vi "CP FES Walking.vi"() -> ()   [LabVIEW 2019]
uses:
  Lee Lab/CP FES Walking 2018/Code/Working/LabVIEW/Controls/Messages/Timer Messages.ctl
  Controls/Messages/CP FES Message.ctl
  <extravilib>/ChannelInstances/Messenger-t'Timer Messages.ctl'.lvlib
  Controls/Protocol Interval.ctl
  Lee Lab/CP FES Walking 2018/Code/Working/LabVIEW/Controls/States/Timer States.ctl
  <extravilib>/ChannelInstances/Event Messenger-bool.lvlib
  Controls/States/CP FES State.ctl
  Controls/Stim Interval Mode.ctl
  <extravilib>/ChannelInstances/Event Messenger-bool/Event Data.ctl
  Controls/Timer Data for timer.ctl
  Controls/Stimulator Mode.ctl
  Controls/Type Defs/Stimulator Control.ctl
  Controls/Type Defs/Stimulator Controls.ctl
  Controls/Interval on-off indicator.ctl
  Controls/Interval Array.ctl
  Controls/Protocol Cluster.ctl
  Controls/APDM Init Cluster.ctl
  Controls/GPD Side Parameters.ctl
  Controls/Stim off-half-ful.ctl
  Controls/Type Defs/Stim Parameters.ctl
  Controls/Subject Params.ctl
  Controls/CP FES Walking Data.ctl
  Controls/Subject.ctl
  Version 2/States/Protocol Timer States.ctl
  Version 2/Data Type Defs/Stim Status.ctl
  Version 2/Data Type Defs/Pulse Mode (array).ctl
  Version 2/Data Type Defs/Stim Update Data.ctl
  Version 2/Data Type Defs/Stim Init Data.ctl
  Version 2/Data Type Defs/Stim Open Data.ctl
  Version 2/Data Type Defs/Stimulator.ctl
  Controls/GPD Parameter Names.ctl
  Controls/APDM Control.ctl
  Controls/Gyro Control.ctl
  Controls/Gyro Controls.ctl
panel:
  in  "View Edit Params":bool
  in  "Thresholding":bool
  in  "Param Ctrls":T1
  out "Iteration Time (ms)":u32
  out "New remaining session time":u32
  out "New time elapsed in current iteration 2":u32
  out "New time to next interval 2":u32
  out "Current interval index 2":u32
  out "Timer State":T2(ring)
  in  "Subject":T3 items=["", "Subject 1", "Subject 2", "Subject 3", "Subject 4", "Subject 5", "Subject 6", "Subject 7", "Subject 8", "Subject 9", "Subject 10", "Subject 11", "Subject 12", "Subject 13", "Subject 14", "Subject 15", "Subject 16", "Subject 17", "Subject 18", "Subject 19", "Subject 20", "Subject 21", "Subject 22", "Subject 23", "Subject 24", "Subject 25", "Subject 26", "Subject 27", "Subject 28", "Subject 29", "Subject 30", "Subject 31", "Subject 32", "Subject 33", "Subject 34", "Subject 35", "Subject 36", "Subject 37", "Subject 38", "Subject 39"]
  in  "Tab Control":T4(tab)
  in  "APDM Hardware":T5
  in  "Protocol":T8={"Active Interval"=[], "Protocol"=[{"Interval Type"=enum."Walk", "Duration"=20.0, " Mode"=enum."Stim", "Alt Period"=0.0}, {"Interval Type"=enum."Rest", "Duration"=20.0, " Mode"=enum."No Stim", "Alt Period"=0.0}, {"Interval Type"=enum."Walk", "Duration"=20.0, " Mode"=enum."Stim", "Alt Period"=0.0}, {"Interval Type"=enum."Rest", "Duration"=20.0, " Mode"=enum."No Stim", "Alt Period"=0.0}, {"Interval Type"=enum."Walk", "Duration"=20.0, " Mode"=enum."Stim", "Alt Period"=0.0}, {"Interval Type"=enum."Rest", "Duration"=20.0, " Mode"=enum."No Stim", "Alt Period"=0.0}, {"Interval Type"=enum."Walk", "Duration"=20.0, " Mode"=enum."Stim", "Alt Period"=0.0}, {"Interval Type"=enum."Rest", "Duration"=20.0, " Mode"=enum."No Stim", "Alt Period"=0.0}, {"Interval Type"=enum."Walk", "Duration"=20.0, " Mode"=enum."Alternating", "Alt Period"=0.0}]}
  in  "Stimulators":T13={"Cluster"={"String 5"="Side", "String"="Stimulator Name", "String 2"="OK", "String 3"="Mode", "String 4"="Timeout (ms)"}, "Left Stimulator Control"={"Side"=enum."Left", "Name"="", "Open"=FALSE, " Mode"="LIVE", "Visa Timeout"=50.0}, "Right Stimulator Control"={"Side"=enum."Right", "Name"="", "Open"=FALSE, " Mode"="LIVE", "Visa Timeout"=50.0}}
  out "GPD Parameter Names":T16=["% Cycle Delay", "Min % Cycle LR to ISw ", "Min % Cycle LR to MSw", "Min % Cycle LR to TSw", "Min % Cycle ISw to MSw", "Min % Cycle TSw to LR", "Max % Cycle TSw to LR", "LR Min Gyro Z Threshold", "LR Min Gyro Z Width", "ISw Peak Threshold", "ISw Peak Width (ms)", "TSw Valley Threshold", "TSw Valley Width (ms)", "Max Cycle Time (s)", "Mean Computation Window"]
  out "GPD Params Display":T18={"Left GPD Params"={"% Cycle Delay"=75.0, "Min % Cycle LR to ISw "=55.0, "Min % Cycle LR to MSw"=50.0, "Min % Cycle LR to TSw"=75.0, "Max % Cycle ISw to MSw"=25.0, "Min % Cycle TSw to LR"=2.5, "Max % Cycle TSw to LR"=75.0, "LR Min Gyro Z Threshold"=-0.3, "LR Min Gyro Z Width"=230.0, "ISw Peak Threshold"=0.6, "ISw Peak Width"=55.0, "TSw Valley Threshold"=-0.5, "TSw Valley Width (ms)"=55.0, "Max Cycle Time (s)"=1.3, "Mean Computation Window"=10.0, "CP subject?"=FALSE}, "Right GPD Params"={"% Cycle Delay"=75.0, "Min % Cycle LR to ISw "=55.0, "Min % Cycle LR to MSw"=50.0, "Min % Cycle LR to TSw"=75.0, "Max % Cycle ISw to MSw"=25.0, "Min % Cycle TSw to LR"=2.5, "Max % Cycle TSw to LR"=75.0, "LR Min Gyro Z Threshold"=-0.3, "LR Min Gyro Z Width"=230.0, "ISw Peak Threshold"=0.6, "ISw Peak Width"=55.0, "TSw Valley Threshold"=-0.5, "TSw Valley Width (ms)"=55.0, "Max Cycle Time (s)"=1.3, "Mean Computation Window"=10.0, "CP subject?"=FALSE}}
  out "Parameters File":string
  out "Stim Params Display":T21
  out "Parameters File":string
  in  "Local Default Parameters File":path=path "\\\\win.udel.edu\\PT/Lee Lab/CP FES Walking 2018"
  out "Timer State":T2(ring)
  out "Iteration Time (ms)":u32
  out "New remaining session time":u32
  out "New time elapsed in current iteration":u32
  out "New time to next interval":u32
  out "Current interval index":u32
  in  "Subject Parameters Folder":path=path "\\\\win.udel.edu\\PT/Lee Lab/CP FES Walking 2018/Subject Parameters"
  in  "Gyro Mode":string(combo)="REAL LIVE GYRO"
  out "Source Parameter File":path
  in  "Stop GPD":bool
  in  "Start GPD":bool
  in  "Start Timer":bool
  in  "Reset":bool
  in  "Manual Stim":bool
  in  "Pause":bool
  in  "Stop":bool
  out "Session Time":dbl[unit] caption="Session Time (s)" format="%.1f"
  out "Time to Next Interval":dbl[unit] caption="Interval Time (s)" format="%.1f"
  # "Save new parameters in new file, load latest version every time"
  # "Present list of all saved parameter files"
  # "Add bluetooth app"
  # "Do an APDM hardware check before allowing Start GPD"
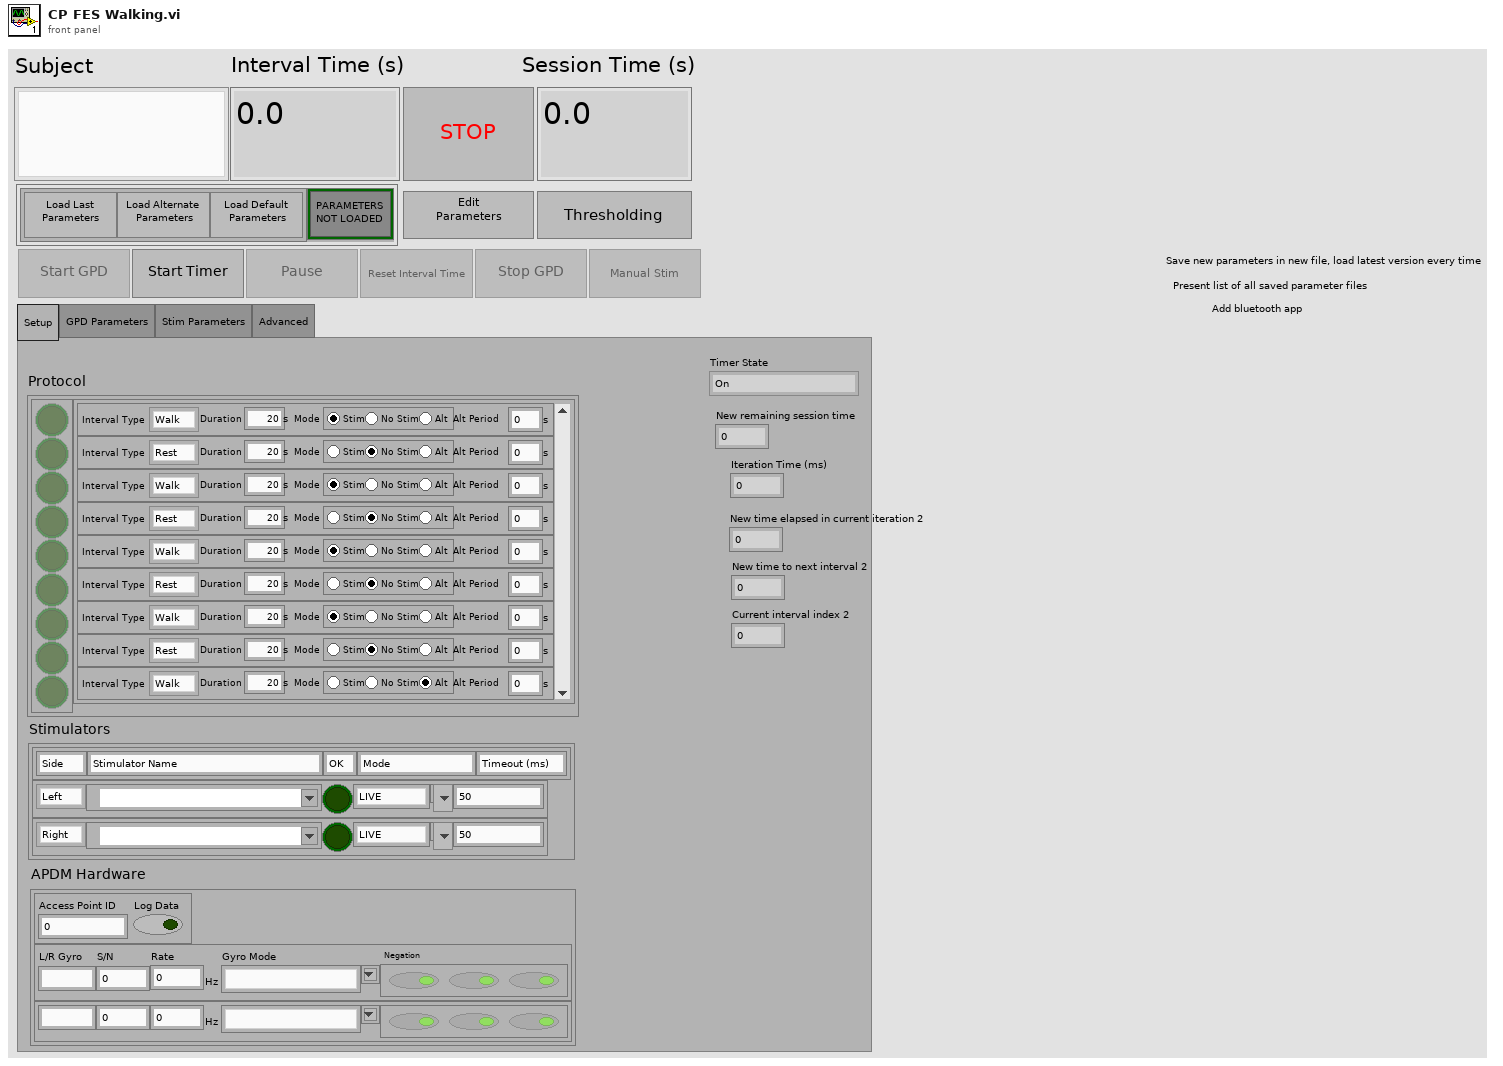
[diagram p1: front panel]
types:
  T1 = cluster{"Param Ctrls":cluster{"Load Last Parameters":bool, "Load Alternate Parameters":bool, "Load Default Parameters":bool}, "Parameters Loaded?":bool}
  T2 = enum16{"On", "Stop", "Pause", "Resume", "Idle", "Initialize"}
  T3 = typedef "Subject.ctl" = u16
  T4 = enum32{"Setup", "GPD Parameters", "Stim Parameters", "Advanced"}
  T5 = typedef "Gyro Controls.ctl" = cluster{"AP Control":T6, "Gyro Control":T7, "Gyro Control 2":T7}
  T6 = typedef "APDM Control.ctl" = cluster{"Access Point ID":u32, "Log Data":bool}
  T7 = typedef "Gyro Control.ctl" = cluster{"L/R":string, "S/N":u32, "Rate":dbl[unit], "Gyro Mode":string, " Negation":bool[]}
  T8 = typedef "Protocol Cluster.ctl" = cluster{"Active Interval":T9[], "Protocol":T10}
  T9 = typedef "Interval on-off indicator.ctl" = bool
  T10 = typedef "Interval Array.ctl" = T11[]
  T11 = typedef "Protocol Interval.ctl" = cluster{"Interval Type":enum16{"Walk", "Rest"}, "Duration":dbl[unit], " Mode":T12, "Alt Period":dbl[unit]}
  T12 = typedef "Stim Interval Mode.ctl" = enum32{"Stim", "No Stim", "Alternating"}
  T13 = typedef "Stimulator Controls.ctl" = cluster{"Cluster":cluster{"String 5":string, "String":string, "String 2":string, "String 3":string, "String 4":string}, "Left Stimulator Control":T14, "Right Stimulator Control":T14}
  T14 = typedef "Stimulator Control.ctl" = cluster{"Side":enum16{"Left", "Right"}, "Name":refnum<visa-resource-name>, "Open":bool, " Mode":T15, "Visa Timeout":dbl}
  T15 = typedef "Stimulator Mode.ctl" = string
  T16 = typedef "GPD Parameter Names.ctl" = string[]
  T17 = typedef "GPD Side Parameters.ctl" = cluster{"% Cycle Delay":dbl, "Min % Cycle LR to ISw ":dbl, "Min % Cycle LR to MSw":dbl, "Min % Cycle LR to TSw":dbl, "Max % Cycle ISw to MSw":dbl, "Min % Cycle TSw to LR":dbl, "Max % Cycle TSw to LR":dbl, "LR Min Gyro Z Threshold":dbl, "LR Min Gyro Z Width":dbl, "ISw Peak Threshold":dbl, "ISw Peak Width":dbl, "TSw Valley Threshold":dbl, "TSw Valley Width (ms)":dbl, "Max Cycle Time (s)":dbl, "Mean Computation Window":dbl, "CP subject?":bool}
  T18 = cluster{"Left GPD Params":T17, "Right GPD Params":T17}
  T19 = typedef "Stim Parameters.ctl" = cluster{"Stim Pattern Values":T20[][], "Pulse Duration":i64[], "Current":i64[]}
  T20 = typedef "Stim off-half-ful.ctl" = enum16{"Off", "Half", "Full"}
  T21 = cluster{"Left Stim Params":T19, "Right Stim Params":T19}
  T22 = typedef "Subject Params.ctl" = cluster{"Subject":T3, "Left GPD Params":T17, "Right GPD Params":T17, "Left Stim Params":T19, "Right Stim Params":T19, "Left Train length":i64[], "Right Train length":i64[]}
  T23 = typedef "APDM Init Cluster.ctl" = cluster{"Log Data":bool, "Gyro Mode":string, "Left  OPAL ID":u32, "Right OPAL ID":u32, "Access Point ID":u32}
  T24 = cluster{"Subject":u16, "Subject Parameter File":path, "Subject Parameters":T22, "Current Interval Idx":i32, "Protocol":T8, "Stimulator Controls":T13, "Stim Protocol Log File":path, "APDM Init Cluster":T23}
  T25 = cluster{"Session Over":refnum<event-registration>, "Interval Over":refnum<event-registration>}
  T26 = typedef "CP FES Message.ctl" = cluster{"State":T27, "Data":variant}
  T27 = typedef "CP FES State.ctl" = enum16{"On", "Stop", "Idle", "Initialize", "Manual", "Stim On", "Stim Off", "Start Timer", "Pause", "Resume", "Reset"}
  T28 = enum8{"Enabled", "Disabled", "Disabled and Grayed Out"}
  T29 = typedef "Timer Data for timer.ctl" = cluster{"Protocol Timer State":T30, "Remaining session time":dbl[unit], "Curent interval duration":dbl[unit], "Time of last iteration":dbl[unit], "Time elapsed in current iteration":dbl[unit], "Current interval indicator":bool[], "Current interval index":u32, "Time to next interval":dbl[unit], "Protocol":T11[]}
  T30 = typedef "Protocol Timer States.ctl" = enum16{"Initialize", "Start", "Advance", "Stop", "Pause", "Resume", "Reset"}
  T31 = typedef "Timer Messages.ctl" = cluster{"Message":T32, "Data":variant}
  T32 = typedef "Timer States.ctl" = enum16{"On", "Stop", "Pause", "Resume", "Idle", "Initialize", "Transition", "Reset", "Start"}
  T33 = typedef "Messenger-t'Timer Messages.ctl'.lvlib/))Channel.ctl" = refnum<queue>
  T34 = typedef "Event Messenger-bool.lvlib/))Channel.ctl" = refnum<queue>
  T35 = typedef "Protocol Cluster.ctl" = cluster{"Active Interval":T9[], "Protocol":T36}
  T36 = typedef "Interval Array.ctl" = T37[]
  T37 = typedef "Protocol Interval.ctl" = cluster{"Interval Type":enum16{"Walk", "Rest"}, "Duration":dbl, "Stim Mode":T12, "Alt Period":dbl}
  T38 = cluster{"Subject Parameter File":path, "Current Interval":T11, "Stim Protocol Log File":path}
  T39 = typedef "CP FES Walking Data.ctl" = cluster{"Subject":u16, "Subject Parameter File":path, "Subject Parameters":T22, "Current Interval Idx":i32, "Protocol":T8, "Stim Protocol Log File":path, "APDM Init Cluster":T23, "Stimulators":T40[]}
  T40 = typedef "Stimulator.ctl" = cluster{"Stim Open Data":T41, "Stim Init Data":T42, "Stim Update Data":T43, "Stim Status":T45}
  T41 = typedef "Stim Open Data.ctl" = cluster{"Name":refnum<visa-resource-name>, "Mode":enum16{"LIVE", "SIM"}, "Visa Timeout":u32}
  T42 = typedef "Stim Init Data.ctl" = cluster{"Frequency":dbl, "N Factor":u8, "D/T Int":dbl, "Active Channels":bool[], "LF Channels":bool[]}
  T43 = typedef "Stim Update Data.ctl" = cluster{"Pulse Mode":T44, "Current":u32[], "Pulse Dur":u32[]}
  T44 = typedef "Pulse Mode (array).ctl" = enum16{"Single", "Doublet", "Triplet"}[]
  T45 = typedef "Stim Status.ctl" = cluster{"Open":bool, "On":bool}
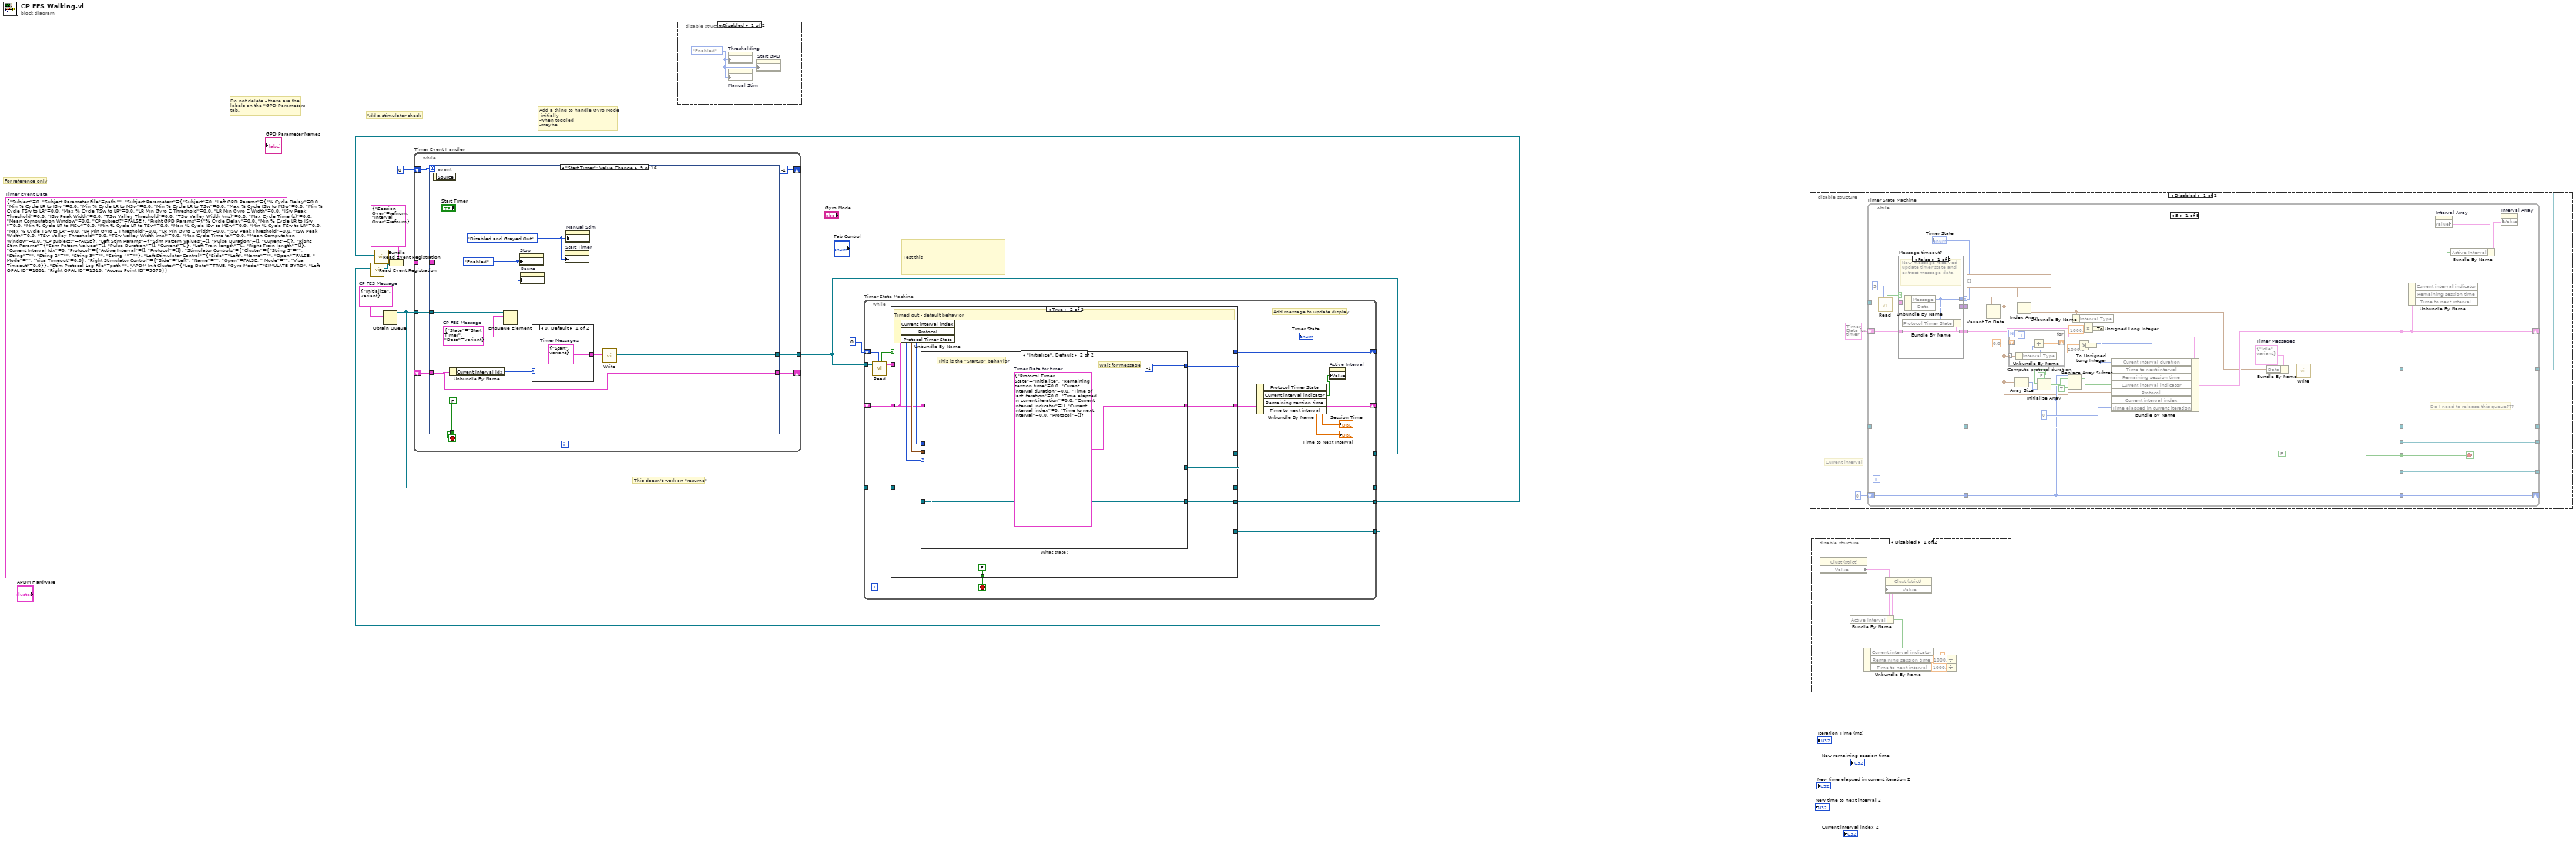
[diagram p0: block diagram]
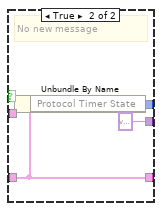
[diagram p3: hidden frame]
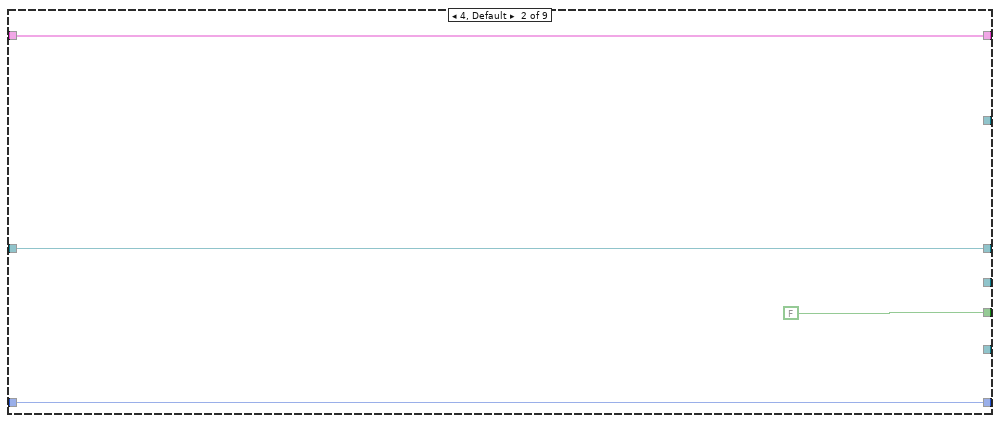
[diagram p4: hidden frame]
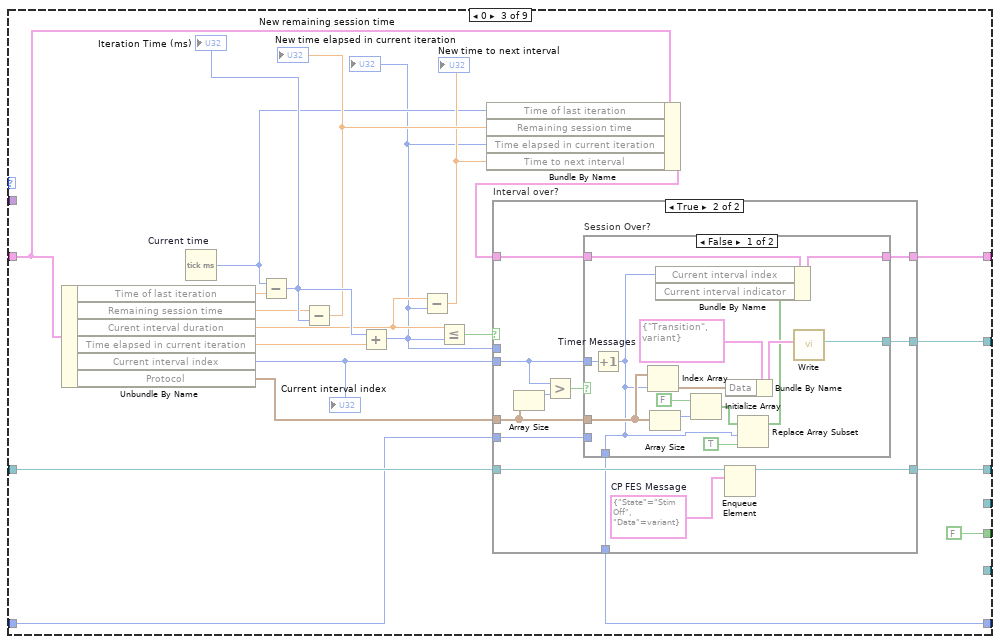
[diagram p5: hidden frame]
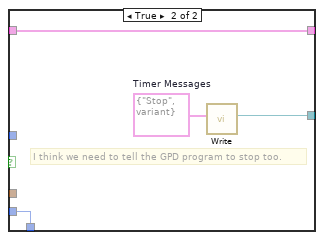
[diagram p7: hidden frame]
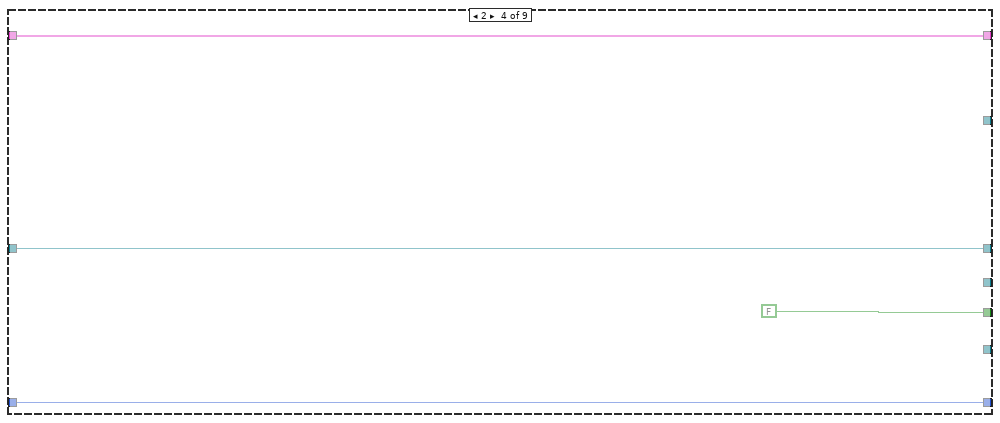
[diagram p8: hidden frame]
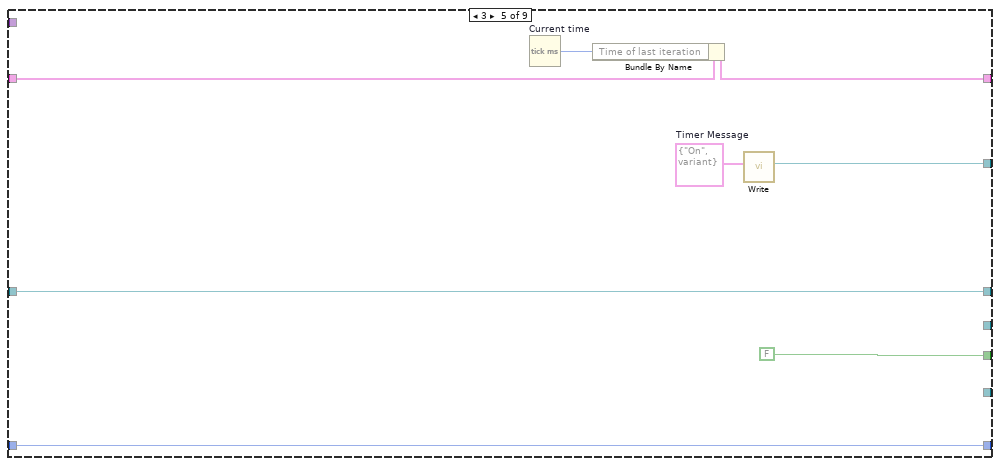
[diagram p9: hidden frame]
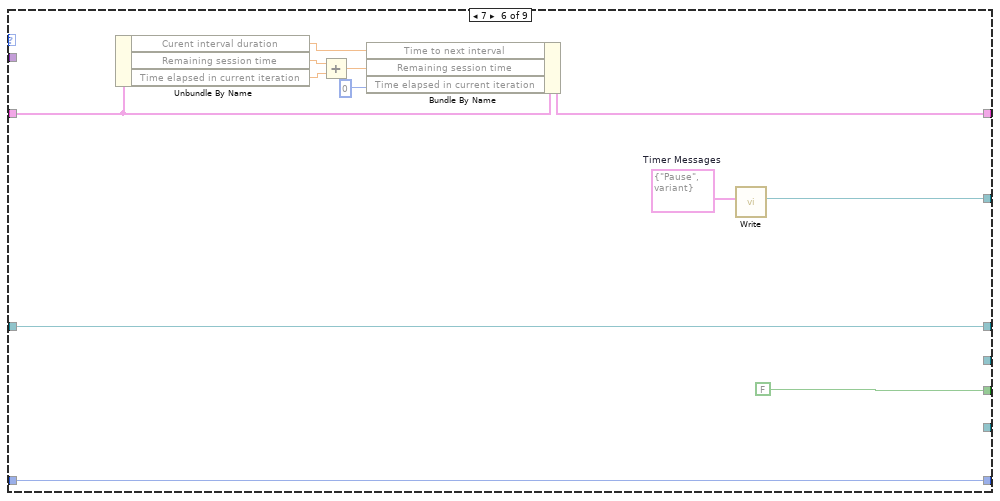
[diagram p10: hidden frame]
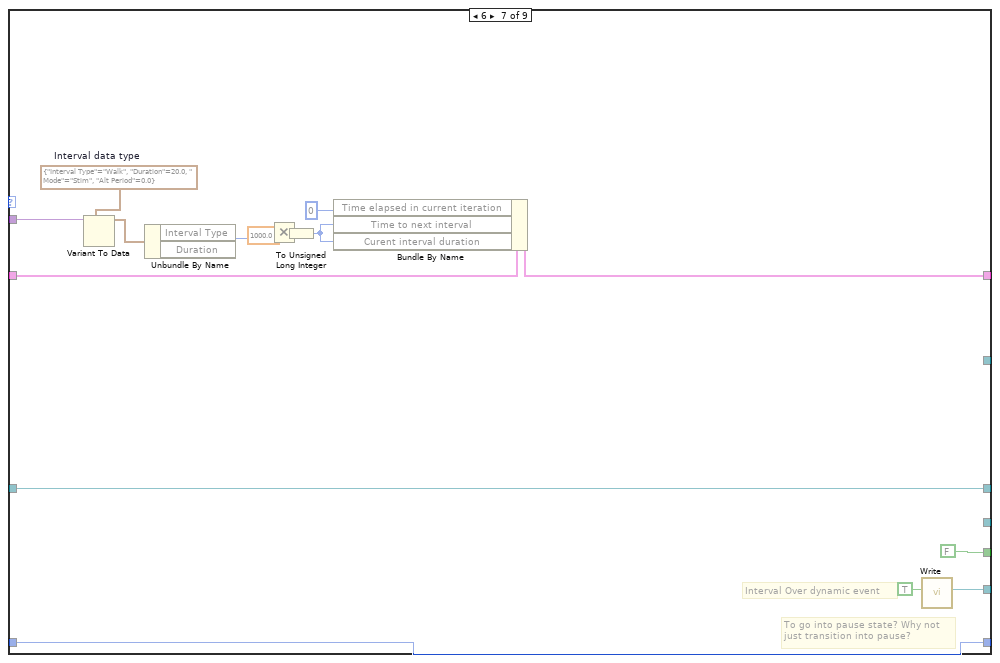
[diagram p11: hidden frame]
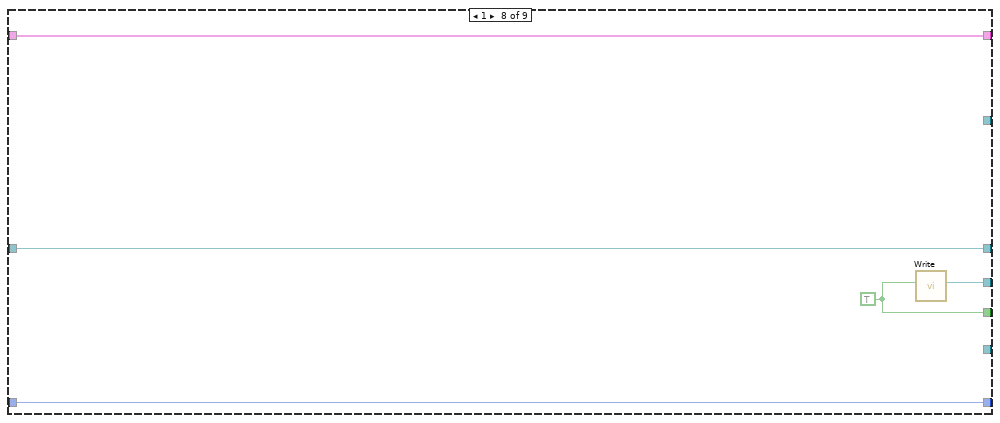
[diagram p12: hidden frame]
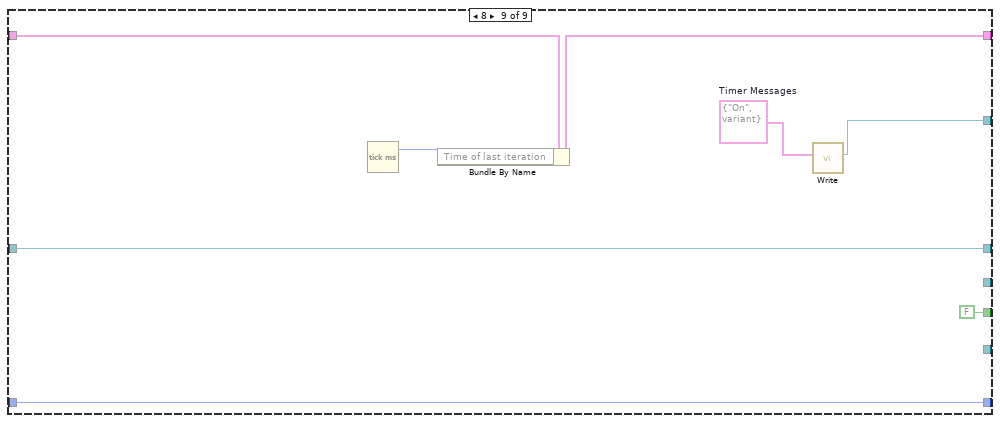
[diagram p13: hidden frame]
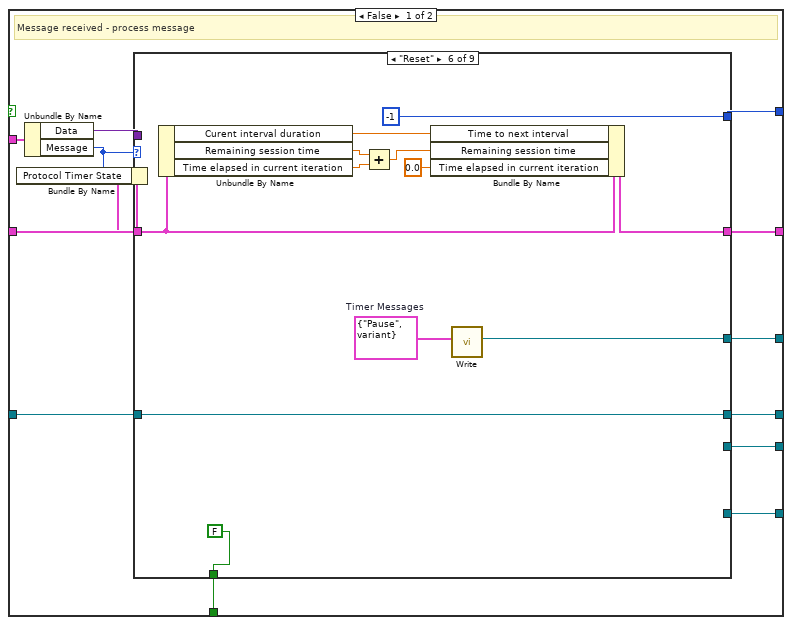
[diagram p16: hidden frame]
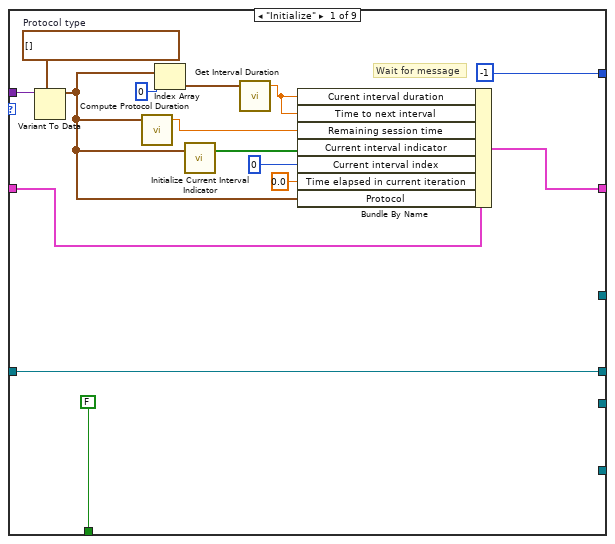
[diagram p17: hidden frame]
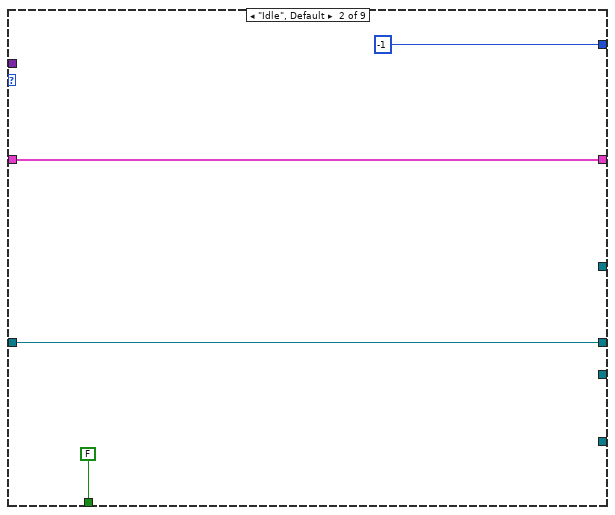
[diagram p18: hidden frame]
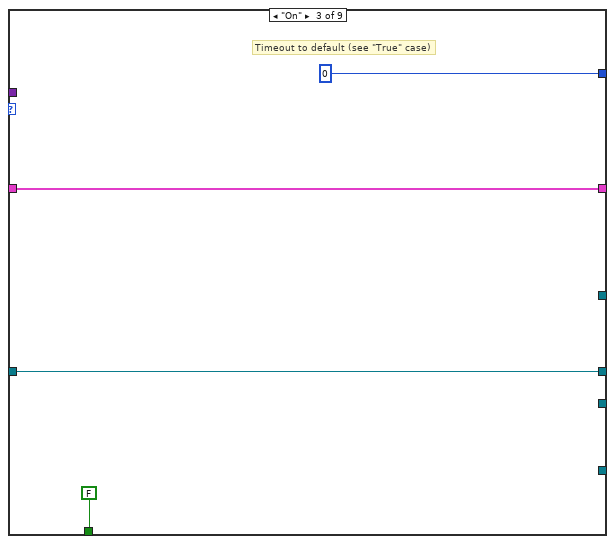
[diagram p19: hidden frame]
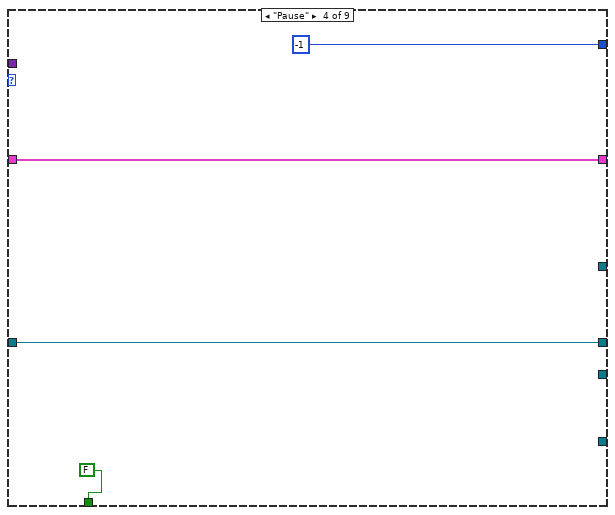
[diagram p20: hidden frame]
diagram:
  (unwired) T24 {"Subject"=0, "Subject Parameter File"=path "", "Subject Parameters"={"Subject"=0, "Left GPD Params"={"% Cycle Delay"=0.0, "Min % Cycle LR to ISw "=0.0, "Min % Cycle LR to MSw"=0.0, "Min % Cycle LR to TSw"=0.0, "Max % Cycle ISw to MSw"=0.0, "Min % Cycle TSw to LR"=0.0, "Max % Cycle TSw to LR"=0.0, "LR Min Gyro Z Threshold"=0.0, "LR Min Gyro Z Width"=0.0, "ISw Peak Threshold"=0.0, "ISw Peak Width"=0.0, "TSw Valley Threshold"=0.0, "TSw Valley Width (ms)"=0.0, "Max Cycle Time (s)"=0.0, "Mean Computation Window"=0.0, "CP subject?"=FALSE}, "Right GPD Params"={"% Cycle Delay"=0.0, "Min % Cycle LR to ISw "=0.0, "Min % Cycle LR to MSw"=0.0, "Min % Cycle LR to TSw"=0.0, "Max % Cycle ISw to MSw"=0.0, "Min % Cycle TSw to LR"=0.0, "Max % Cycle TSw to LR"=0.0, "LR Min Gyro Z Threshold"=0.0, "LR Min Gyro Z Width"=0.0, "ISw Peak Threshold"=0.0, "ISw Peak Width"=0.0, "TSw Valley Threshold"=0.0, "TSw Valley Width (ms)"=0.0, "Max Cycle Time (s)"=0.0, "Mean Computation Window"=0.0, "CP subject?"=FALSE}, "Left Stim Params"={"Stim Pattern Values"=[], "Pulse Duration"=[], "Current"=[]}, "Right Stim Params"={"Stim Pattern Values"=[], "Pulse Duration"=[], "Current"=[]}, "Left Train length"=[], "Right Train length"=[]}, "Current Interval Idx"=0, "Protocol"={"Active Interval"=[], "Protocol"=[]}, "Stimulator Controls"={"Cluster"={"String 5"="", "String"="", "String 2"="", "String 3"="", "String 4"=""}, "Left Stimulator Control"={"Side"=enum."Left", "Name"="", "Open"=FALSE, " Mode"="", "Visa Timeout"=0.0}, "Right Stimulator Control"={"Side"=enum."Left", "Name"="", "Open"=FALSE, " Mode"="", "Visa Timeout"=0.0}}, "Stim Protocol Log File"=path "", "APDM Init Cluster"={"Log Data"=TRUE, "Gyro Mode"="SIMULATE GYRO", "Left  OPAL ID"=1801, "Right OPAL ID"=1510, "Access Point ID"=9370}}  # Timer Event Data
  w11 = T26 {"State"=enum."Initialize", "Data"=variant}  # CP FES Message
  # "Do not delete - these are the\nlabels on the \"GPD Parameters\ntab."
  # "For reference only"
  # "This doesn't work on \"resume\""
  # "Test this"
  # "Add a thing to handle Gyro Mode\n-initially\n-when toggled\n-maybe"
  # "Add a stimulator check"
  n1 = Obtain Queue(element data type=w11) -> (queue out=w1:refnum<queue>)  [unwired: 4 in, 2 out]
  n2 = disable-structure shown="Disabled" {
    frame Disabled {
      w12 = T28."Enabled" ("Disabled")
      n3 = property on="Thresholding" class="Bool"("DisabledEnum"=w12) -> ()  [unwired: 2 in, 2 out]
      n4 = property on="Manual Stim" class="Bool (strict)"("DisabledEnum"=w12) -> ()  [unwired: 2 in, 2 out]
      n5 = property on="Start GPD" class="Bool"("DisabledEnum"=w12) -> ()  [unwired: 2 in, 2 out]
    }
    frame Enabled {
    }
  }
  n6 = disable-structure shown="Disabled" {
    frame Disabled {
      # "Current interval"
      n7 = while "Timer State Machine" {
        tunnel: w13 -> [w37]
        tunnel: [w32] -> w13
        shift-right: [w28] -> _
        shift-left: T29 {"Protocol Timer State"=enum."Initialize", "Remaining session time"=0.0, "Curent interval duration"=0.0, "Time of last iteration"=0.0, "Time elapsed in current iteration"=0.0, "Current interval indicator"=[], "Current interval index"=0, "Time to next interval"=0.0, "Protocol"=[]} -> [w30]
        tunnel: [w26] -> _
        tunnel: [w25] -> w15
        tunnel: [w24] -> _
        tunnel: [w23] -> _
        shift-right: [w22] -> _
        shift-left: u32 0 -> [w21]
        stop <- w34 stop-if-true
        # "Do I need to release this queue???"
        n8 = call <extravilib>:"Read.vi"("timeout in ms (-1)"=5, "channel"=w37) -> ("element"=w36:T31, "timedout?"=w31:bool)  [unwired: 6 in, 2 out]
        n9 = case "Message timeout?" shown="False" w31 {
          tunnel: w36 -> [w42 _]
          tunnel: [w40 w43] -> w35
          tunnel: [w41 variant ("Data")] -> w33
          tunnel: w30 -> [w39 w44]
          tunnel: [w38 w44] -> w29
          frame False {
            # "New message received - update timer state and extract message data"
            n10 = Unbundle By Name(w42) -> ("Message"=w40:T32, "Data"=w41:variant)
            n11 = Bundle By Name(cluster=w39, "Protocol Timer State"=w40) -> (w38:T29)
          }
          frame True {
            # "No new message"
            n12 = Unbundle By Name(w44) -> ("Protocol Timer State"=w43:T30)
          }
        }
        "Timer State" <- w35
        n13 = case shown="5" w35 {
          tunnel: [FALSE FALSE FALSE FALSE FALSE FALSE FALSE w177 FALSE] -> w34
          tunnel: w33 -> [w69 _ _ _ _ _ w172 _ _]
          tunnel: [w67 _ w100 _ w144 w156 _ _ w183] -> w32
          tunnel: w29 -> [w58 w79 w92 w137 w143 w153 w167 w178 w185]
          tunnel: [w53 w79 w88 w137 w141 w150 w166 w178 w184] -> w28
          tunnel: [_ _ _ _ _ _ _ w176 _] -> w26
          tunnel: w25 -> [w50 w78 w86 w136 w140 w149 w160 w175 w181]
          tunnel: [w50 w78 w83 w136 w140 w149 w160 w175 w181] -> w24
          tunnel: [_ _ _ _ _ _ w161 _ _] -> w23
          tunnel: [w48 w77 w82 w135 w139 w148 w159 w174 w180] -> w22
          tunnel: w21 -> [w48 w77 w81 w135 w139 w148 w159 w174 w180]
          frame 5 {
            w66 = T31 {"Message"=enum."Idle", "Data"=variant}  # Timer Messages
            n14 = Variant To Data(type=T11[] [], Variant=w69) -> (data=w46:T11[])  [unwired: 1 in, 1 out]
            n15 = for "Compute protocol duration" {
              shift-right: [w75] -> w59
              shift-left: 0.0 -> [w76]
              tunnel: w46 -> [w74] mode=indexing
              n16 = Unbundle By Name(w74) -> ("Interval Type"=w73:enum16{"Walk", "Rest"})
              n17 = Add(x=w76, y=w73) -> (x+y=w75:dbl)
            }
            n18 = Array Size(array=w46) -> (size(s)=w71:i32)
            n19 = Index Array(array=w46) -> (element=w47:T11)  [unwired: 1 in]
            n20 = Initialize Array(FALSE, w71) -> (w55:bool[])
            n21 = Replace Array Subset(array=w55, new element=TRUE ("new element/subarray"), index=w48) -> (w52:bool[])
            n22 = Unbundle By Name(w47) -> ("Interval Type"=w64:enum16{"Walk", "Rest"})
            n23 = Multiply(x=w59, y=1000.0) -> (x*y=w60:dbl)
            n24 = Multiply(x=w64, y=1000.0) -> (x*y=w62:dbl)
            n25 = To Unsigned Long Integer(number=w60) -> (unsigned 32bit integer=w54:u32)
            n26 = To Unsigned Long Integer(number=w62) -> (unsigned 32bit integer=w56:u32)
            n27 = Bundle By Name(cluster=w58, "Curent interval duration"=w56, "Time to next interval"=w56, "Remaining session time"=w54, "Current interval indicator"=w52, "Protocol"=w46, "Current interval index"=w48, "Time elapsed in current iteration"=u32 0) -> (w53:T29)
            n28 = Bundle By Name(cluster=w66, "Data"=w47) -> (w65:T31)
            n29 = call <extravilib>:"Write.vi"("element"=w65) -> ("channel"=w67:T33)  [unwired: 8 in, 2 out]
          }
          frame 4, Default {
          }
          frame 0 {
            n30 = Unbundle By Name(w92) -> ("Time of last iteration"=w96:dbl[unit], "Remaining session time"=w97:dbl[unit], "Curent interval duration"=w94:dbl[unit], "Time elapsed in current iteration"=w85:dbl[unit], "Current interval index"=w95:u32, "Protocol"=w93:T11[])
            "Current interval index" <- w95
            n31 = Tick Count (ms) "Current time"() -> (millisecond timer value=w87:u32)
            n32 = Subtract(x=w87, y=w96) -> (x-y=w98:u32)
            "Iteration Time (ms)" <- w98
            n33 = Subtract(x=w97, y=w98) -> (x-y=w91:dbl[unit])
            "New remaining session time" <- w91
            n34 = Add(x=w98, y=w85) -> (x+y=w84:u32)
            "New time elapsed in current iteration" <- w84
            n35 = Subtract(x=w94, y=w84) -> (x-y=w90:dbl[unit])
            "New time to next interval" <- w90
            n36 = Less Or Equal?(x=w94, y=w84) -> (x <= y?=w101:bool)
            n37 = Bundle By Name(cluster=w92, "Time of last iteration"=w87, "Remaining session time"=w91, "Time elapsed in current iteration"=w84, "Time to next interval"=w90) -> (w89:T29)
            n38 = case "Interval over?" shown="True" w101 {
              tunnel: w95 -> [_ w114]
              tunnel: [_ w116] -> w100
              tunnel: w93 -> [_ w112]
              tunnel: w89 -> [w104 w111]
              tunnel: [w104 w110] -> w88
              tunnel: w84 -> [_ _]
              tunnel: w86 -> [w103 w108]
              tunnel: [w103 w107] -> w83
              tunnel: [w102 w106] -> w82
              tunnel: w81 -> [w102 w105]
              frame False {
                # "Why don't we need to send On to self here?"
              }
              frame True {
                w109 = T26 {"State"=enum."Stim Off", "Data"=variant}  # CP FES Message
                n39 = Array Size(array=w112) -> (size(s)=w115:i32)
                n40 = Greater?(x=w114, y=w115) -> (0:w113:bool)
                n41 = case "Session Over?" shown="False" w113 {
                  tunnel: w114 -> [w118 _]
                  tunnel: [w130 w134] -> w116
                  tunnel: w112 -> [w122 _]
                  tunnel: w111 -> [w121 w132]
                  tunnel: [w120 w132] -> w110
                  tunnel: [w117 w131] -> w106
                  tunnel: w105 -> [_ w131]
                  frame False {
                    w129 = T31 {"Message"=enum."Transition", "Data"=variant}  # Timer Messages
                    n42 = Increment(x=w118) -> (x+1=w117:u32)
                    n43 = Index Array(array=w122, index=w117) -> (element=w127:T11)
                    n44 = Array Size(array=w122) -> (size(s)=w124:i32)
                    n45 = Initialize Array(FALSE ("element"), w124) -> (w126:bool[])
                    n46 = Bundle By Name(cluster=w129, "Data"=w127) -> (w128:T31)
                    n47 = Replace Array Subset(array=w126, new element=TRUE ("new element/subarray"), index=w117) -> (w119:bool[])
                    n48 = Bundle By Name(cluster=w121, "Current interval index"=w117, "Current interval indicator"=w119) -> (w120:T29)
                    n49 = call <extravilib>:"Write.vi"("element"=w128) -> ("channel"=w130:T33)  [unwired: 8 in, 2 out]
                  }
                  frame True {
                    w133 = T31 {"Message"=enum."Stop", "Data"=variant}  # Timer Messages
                    # "I think we need to tell the GPD program to stop too."
                    n50 = call <extravilib>:"Write.vi"("element"=w133) -> ("channel"=w134:T33)  [unwired: 8 in, 2 out]
                  }
                }
                n51 = Enqueue Element(queue=w108, element=w109) -> (queue out=w107:refnum<queue>)  [unwired: 2 in, 2 out]
              }
            }
          }
          frame 2 {
          }
          frame 3 {
            w145 = T31 {"Message"=enum."On", "Data"=variant}  # Timer Message
            n52 = Tick Count (ms) "Current time"() -> (millisecond timer value=w142:u32)
            n53 = Bundle By Name(cluster=w143, "Time of last iteration"=w142) -> (w141:T29)
            n54 = call <extravilib>:"Write.vi"("element"=w145) -> ("channel"=w144:T33)  [unwired: 8 in, 2 out]
          }
          frame 7 {
            w157 = T31 {"Message"=enum."Pause", "Data"=variant}  # Timer Messages
            n55 = Unbundle By Name(w153) -> ("Curent interval duration"=w147:dbl[unit], "Remaining session time"=w155:dbl[unit], "Time elapsed in current iteration"=w154:dbl[unit])
            n56 = Add(x=w155, y=w154) -> (x+y=w152:dbl[unit])
            n57 = Bundle By Name(cluster=w153, "Time to next interval"=w147, "Remaining session time"=w152, "Time elapsed in current iteration"=u32 0) -> (w150:T29)
            n58 = call <extravilib>:"Write.vi"("element"=w157) -> ("channel"=w156:T33)  [unwired: 8 in, 2 out]
          }
          frame 6 {
            w173 = T11 {"Interval Type"=enum."Walk", "Duration"=20.0, " Mode"=enum."Stim", "Alt Period"=0.0}  # Interval data type
            # "To go into pause state? Why not\njust transition into pause?"
            # "Interval Over dynamic event"
            n59 = Variant To Data(type=w173, Variant=w172) -> (data=w163:T11)  [unwired: 1 in, 1 out]
            n60 = Unbundle By Name(w163) -> ("Interval Type"=w171:enum16{"Walk", "Rest"})  [unwired: 1 out]
            n61 = Multiply(x=w171, y=1000.0) -> (x*y=w169:dbl)
            n62 = To Unsigned Long Integer(number=w169) -> (unsigned 32bit integer=w164:u32)
            n63 = Bundle By Name(cluster=w167, "Time elapsed in current iteration"=u32 0, "Time to next interval"=w164, "Curent interval duration"=w164) -> (w166:T29)
            n64 = call <extravilib>:"Write.vi"("element"=TRUE) -> ("channel"=w161:T34)  [unwired: 9 in, 1 out]
          }
          frame 1 {
            w177 = TRUE
            n65 = call <extravilib>:"Write.vi"("element"=w177) -> ("channel"=w176:T34)  [unwired: 9 in, 1 out]
          }
          frame 8 {
            w182 = T31 {"Message"=enum."On", "Data"=variant}  # Timer Messages
            n66 = Tick Count (ms)() -> (millisecond timer value=w186:u32)
            n67 = Bundle By Name(cluster=w185, "Time of last iteration"=w186) -> (w184:T29)
            n68 = call <extravilib>:"Write.vi"("element"=w182) -> ("channel"=w183:T33)  [unwired: 8 in, 2 out]
          }
        }
        n69 = Unbundle By Name(w28) -> ("Current interval indicator"=w19:bool[], "Remaining session time"=w27:dbl[unit])  [unwired: 1 out]
        n70 = property on="Interval Array" class="Clust (strict)"() -> ("Value"=w17:T8)  [unwired: 2 in, 2 out]
        n71 = Bundle By Name(cluster=w17, "Active Interval"=w19) -> (w18:T8)
        n72 = property on="Interval Array" class="Clust (strict)"("Value"=w18) -> ()  [unwired: 2 in, 2 out]
      }
    }
    frame Enabled {
    }
  }
  n73 = disable-structure shown="Disabled" {
    frame Disabled {
      n74 = property on="Property Node" class="Clust (strict)"() -> ("Value"=w193:T35)  [unwired: 2 in, 2 out]
      n75 = Unbundle By Name() -> ("Current interval indicator"=w191:bool[], "Remaining session time"=w189:u32, "Time to next interval"=w190:u32)  [unwired: 1 in]
      n76 = Bundle By Name(cluster=w193, "Active Interval"=w191) -> (w192:T35)
      n77 = property on="Property Node" class="Clust (strict)"("Value"=w192) -> ()  [unwired: 2 in, 2 out]
      n78 = Divide(x=w189, y=1000.0) -> ()  [unwired: 1 out]
      n79 = Divide(x=w190, y=1000.0) -> ()  [unwired: 1 out]
    }
    frame Enabled {
    }
  }
  n80 = call <extravilib>:"Read Event Registration.vi"("channel"=w3) -> ("event registration refnum"=w9:refnum<event-registration>)  [unwired: 10 in]
  n81 = call <extravilib>:"Read Event Registration.vi"("channel"=w4) -> ("event registration refnum"=w10:refnum<event-registration>)  [unwired: 10 in]
  n82 = Bundle(cluster=T25 {"Session Over"=refnum, "Interval Over"=refnum}, "Session Over"=w10, "Interval Over"=w9) -> (w8:T25)
  n83 = while "Timer Event Handler" {
    tunnel: w1 -> [w201]
    tunnel: [w200] -> w2
    tunnel: w8 -> [w198]
    shift-right: [-1] -> _
    shift-left: 0 -> [w197]
    shift-right: [w195] -> _
    shift-left: _ -> [w194]
    stop <- w199 stop-if-true
    n84 = event shown="[8] \"Start Timer\": Value Change" {
      selector: w198 -> [_ _ _ _ _ _ _ _ _ _ _ _ _ _ _ _]
      dyn-events: _ -> [_ _ _ _ _ _ _ _ _ _ _ _ _ _ _ _]
      timeout: w197 -> [_ _ _ _ _ _ _ _ _ _ _ _ _ _ _ _]
      tunnel: w201 -> [_ _ _ _ _ _ _ w310 w324 w341 w351 w361 w366 w384 w387 _]
      tunnel: [w202 _ _ _ _ _ w277 _ w330 w335 w355 w358 _ _ _ w397] -> w200
      tunnel: [FALSE FALSE FALSE FALSE FALSE FALSE FALSE FALSE FALSE FALSE FALSE TRUE FALSE FALSE TRUE FALSE] -> w199
      tunnel: [w207 w240 w260 w268 w270 w274 w283 w285 w322 w333 w349 w357 w363 w382 w386 w390] -> w195
      tunnel: w194 -> [_ w244 w259 w269 w271 w275 w284 w285 w322 w333 w349 w357 w363 w382 w386 w391]
      event Timeout {
        w206 = T31 {"Message"=enum."Initialize", "Data"=variant}  # Timer Messages
        w211 = T21 {"Left Stim Params"={"Stim Pattern Values"=[], "Pulse Duration"=[], "Current"=[]}, "Right Stim Params"={"Stim Pattern Values"=[], "Pulse Duration"=[], "Current"=[]}}  # Stim Params Display (zeroed)
        w212 = T18 {"Left GPD Params"={"% Cycle Delay"=0.0, "Min % Cycle LR to ISw "=0.0, "Min % Cycle LR to MSw"=0.0, "Min % Cycle LR to TSw"=0.0, "Max % Cycle ISw to MSw"=0.0, "Min % Cycle TSw to LR"=0.0, "Max % Cycle TSw to LR"=0.0, "LR Min Gyro Z Threshold"=0.0, "LR Min Gyro Z Width"=0.0, "ISw Peak Threshold"=0.0, "ISw Peak Width"=0.0, "TSw Valley Threshold"=0.0, "TSw Valley Width (ms)"=0.0, "Max Cycle Time (s)"=0.0, "Mean Computation Window"=0.0, "CP subject?"=FALSE}, "Right GPD Params"={"% Cycle Delay"=0.0, "Min % Cycle LR to ISw "=0.0, "Min % Cycle LR to MSw"=0.0, "Min % Cycle LR to TSw"=0.0, "Max % Cycle ISw to MSw"=0.0, "Min % Cycle TSw to LR"=0.0, "Max % Cycle TSw to LR"=0.0, "LR Min Gyro Z Threshold"=0.0, "LR Min Gyro Z Width"=0.0, "ISw Peak Threshold"=0.0, "ISw Peak Width"=0.0, "TSw Valley Threshold"=0.0, "TSw Valley Width (ms)"=0.0, "Max Cycle Time (s)"=0.0, "Mean Computation Window"=0.0, "CP subject?"=FALSE}}  # GPD Params Display (zeroed)
        w208 = T39 {"Subject"=0, "Subject Parameter File"=path "", "Subject Parameters"={"Subject"=0, "Left GPD Params"={"% Cycle Delay"=75.0, "Min % Cycle LR to ISw "=55.0, "Min % Cycle LR to MSw"=50.0, "Min % Cycle LR to TSw"=75.0, "Max % Cycle ISw to MSw"=10.0, "Min % Cycle TSw to LR"=2.5, "Max % Cycle TSw to LR"=75.0, "LR Min Gyro Z Threshold"=-0.3, "LR Min Gyro Z Width"=230.0, "ISw Peak Threshold"=0.6, "ISw Peak Width"=55.0, "TSw Valley Threshold"=-0.5, "TSw Valley Width (ms)"=55.0, "Max Cycle Time (s)"=1.3, "Mean Computation Window"=10.0, "CP subject?"=FALSE}, "Right GPD Params"={"% Cycle Delay"=75.0, "Min % Cycle LR to ISw "=55.0, "Min % Cycle LR to MSw"=50.0, "Min % Cycle LR to TSw"=75.0, "Max % Cycle ISw to MSw"=10.0, "Min % Cycle TSw to LR"=2.5, "Max % Cycle TSw to LR"=75.0, "LR Min Gyro Z Threshold"=-0.3, "LR Min Gyro Z Width"=230.0, "ISw Peak Threshold"=0.6, "ISw Peak Width"=55.0, "TSw Valley Threshold"=-0.5, "TSw Valley Width (ms)"=55.0, "Max Cycle Time (s)"=1.3, "Mean Computation Window"=10.0, "CP subject?"=FALSE}, "Left Stim Params"={"Stim Pattern Values"=[[enum."Full", enum."Half", enum."Off", enum."Off", enum."Off", enum."Off", enum."Half"], [enum."Full", enum."Off", enum."Off", enum."Off", enum."Off", enum."Half", enum."Half"], [enum."Half", enum."Full", enum."Off", enum."Full", enum."Off", enum."Off", enum."Full"], [enum."Half", enum."Off", enum."Off", enum."Half", enum."Full", enum."Full", enum."Full"], [enum."Off", enum."Full", enum."Half", enum."Half", enum."Off", enum."Off", enum."Off"]], "Pulse Duration"=[20, 200, 200, 200, 200], "Current"=[20, 20, 20, 20, 20]}, "Right Stim Params"={"Stim Pattern Values"=[[enum."Full", enum."Half", enum."Off", enum."Off", enum."Off", enum."Off", enum."Half"], [enum."Full", enum."Off", enum."Off", enum."Off", enum."Off", enum."Half", enum."Half"], [enum."Half", enum."Full", enum."Off", enum."Full", enum."Off", enum."Off", enum."Full"], [enum."Half", enum."Off", enum."Off", enum."Half", enum."Full", enum."Full", enum."Full"], [enum."Off", enum."Full", enum."Half", enum."Half", enum."Off", enum."Off", enum."Off"]], "Pulse Duration"=[200, 200, 200, 200, 200], "Current"=[200, 200, 200, 200, 200]}, "Left Train length"=[300, 300, 300, 300, 300], "Right Train length"=[300, 300, 300, 300, 300]}, "Current Interval Idx"=0, "Protocol"={"Active Interval"=[], "Protocol"=[{"Interval Type"=enum."Walk", "Duration"=20.0, " Mode"=enum."Stim", "Alt Period"=0.0}, {"Interval Type"=enum."Rest", "Duration"=20.0, " Mode"=enum."No Stim", "Alt Period"=0.0}, {"Interval Type"=enum."Walk", "Duration"=20.0, " Mode"=enum."Stim", "Alt Period"=0.0}, {"Interval Type"=enum."Rest", "Duration"=20.0, " Mode"=enum."No Stim", "Alt Period"=0.0}, {"Interval Type"=enum."Walk", "Duration"=20.0, " Mode"=enum."Stim", "Alt Period"=0.0}, {"Interval Type"=enum."Rest", "Duration"=20.0, " Mode"=enum."No Stim", "Alt Period"=0.0}, {"Interval Type"=enum."Walk", "Duration"=20.0, " Mode"=enum."Stim", "Alt Period"=0.0}, {"Interval Type"=enum."Rest", "Duration"=20.0, " Mode"=enum."No Stim", "Alt Period"=0.0}, {"Interval Type"=enum."Walk", "Duration"=20.0, " Mode"=enum."Alternating", "Alt Period"=0.0}]}, "Stim Protocol Log File"=path "", "APDM Init Cluster"={"Log Data"=TRUE, "Gyro Mode"="SIMULATE GYRO", "Left  OPAL ID"=0, "Right OPAL ID"=0, "Access Point ID"=0}, "Stimulators"=[]}  # CP FES Walking Data
        w220 = u16 0 items=["Subject 0", "Subject 1", "Subject 2", "Subject 3", "Subject 4", "Subject 5", "Subject 6", "Subject 7", "Subject 8", "Subject 9", "Subject 10", "Subject 11", "Subject 12", "Subject 13", "Subject 14", "Subject 15", "Subject 16", "Subject 17", "Subject 18", "Subject 19", "Subject 20", "Subject 21", "Subject 22", "Subject 23", "Subject 24", "Subject 25", "Subject 26", "Subject 27", "Subject 28", "Subject 29", "Subject 30", "Subject 31", "Subject 32", "Subject 33", "Subject 34", "Subject 35", "Subject 36", "Subject 37", "Subject 38", "Subject 39", "Subject 40"] ("Subject")
        w222 = 40  # Number of Subjects
        w210 = T28."Disabled and Grayed Out" ("Disabled")
        # "Might be cleaner to load protocol from file"
        # "Set default stimulator controls here"
        # "Initialization"
        n85 = event-data() -> ()  [unwired: 1 in, 1 out]
        n86 = call "Generate Subject Strings.vi"("Number of Subjects"=w222) -> ("Array"=w221:string[])  [unwired: 2 in]
        n87 = call <vilib>:"Application Directory.vi"() -> ("Application Directory"=w216:path)
        n88 = property on="Stop" class="Bool"("DisabledEnum"=T28."Enabled" ("Disabled")) -> ()  [unwired: 2 in, 2 out]
        n89 = Bundle By Name(cluster=w208, "Protocol"="Protocol") -> (w207:T39)
        n90 = property on="Subject" class="Ring (strict)"("Strings []"=w221) -> ()  [unwired: 2 in, 2 out]
        n91 = Build Path(base path=w216, name or relative path="subj_00_params.prm") -> (appended path=w215:path)
        n92 = property on="Local Default Parameters File" class="Path"("Value"=w215) -> ()  [unwired: 2 in, 2 out]
        n93 = disable-structure shown="Disabled" {
          frame Disabled {
            w224 = FALSE
            n94 = property on="Stop" class="Bool"("Value"=w224) -> ()  [unwired: 2 in, 2 out]
            n95 = property on="Start Timer" class="Bool"("Value"=w224) -> ()  [unwired: 2 in, 2 out]
            n96 = property on="Pause" class="Bool (strict)"("Value"=w224) -> ()  [unwired: 2 in, 2 out]
            n97 = property on="Manual Stim" class="Bool (strict)"("Value"=w224) -> ()  [unwired: 2 in, 2 out]
            n98 = property on="Start GPD" class="Bool"("Value"=w224) -> ()  [unwired: 2 in, 2 out]
            n99 = property on="Reset" class="Bool"("Value"=w224) -> ()  [unwired: 2 in, 2 out]
          }
          frame Enabled {
          }
        }
        n100 = property on="Thresholding" class="Bool"("DisabledEnum"=w210) -> ()  [unwired: 2 in, 2 out]
        n101 = property on="Start Timer" class="Bool"("DisabledEnum"=w210) -> ()  [unwired: 2 in, 2 out]
        n102 = property on="View Edit Params" class="Bool"("DisabledEnum"=w210) -> ()  [unwired: 2 in, 2 out]
        n103 = property on="Manual Stim" class="Bool (strict)"("DisabledEnum"=w210) -> ()  [unwired: 2 in, 2 out]
        n104 = property on="Pause" class="Bool (strict)"("DisabledEnum"=w210) -> ()  [unwired: 2 in, 2 out]
        n105 = property on="Start GPD" class="Bool"("DisabledEnum"=w210) -> ()  [unwired: 2 in, 2 out]
        n106 = property on="Subject" class="Ring (strict)"("Value"=w220) -> ()  [unwired: 2 in, 2 out]
        n107 = Unbundle By Name("Protocol") -> ("Protocol"=w203:T10)
        n108 = property on="Source Parameter File" class="Path"("Value"=path "") -> ()  [unwired: 2 in, 2 out]
        n109 = Bundle By Name(cluster=w206, "Data"=w203) -> (w205:T31)
        n110 = property on="GPD Params Display" class="Clust (strict)"("Value"=w212) -> ()  [unwired: 2 in, 2 out]
        n111 = property on="Param Ctrls" class="Clust"("Value"=T1 {"Param Ctrls"={"Load Last Parameters"=FALSE, "Load Alternate Parameters"=FALSE, "Load Default Parameters"=FALSE}, "Parameters Loaded?"=FALSE} ("Param Ctrls"), "DisabledEnum"=T28."Disabled and Grayed Out" ("Disabled")) -> ()  [unwired: 2 in, 2 out]
        n112 = property on="Stim Params Display" class="Clust (strict)"("Value"=w211) -> ()  [unwired: 2 in, 2 out]
        n113 = property on="Stimulators" class="Clust (strict)"("Value"=T13 {"Cluster"={"String 5"="Side", "String"="Stimulator Name", "String 2"="OK", "String 3"="Mode", "String 4"="Timeout (ms)"}, "Left Stimulator Control"={"Side"=enum."Left", "Name"="", "Open"=FALSE, " Mode"="SIMULATED", "Visa Timeout"=50.0}, "Right Stimulator Control"={"Side"=enum."Right", "Name"="", "Open"=FALSE, " Mode"="SIMULATED", "Visa Timeout"=50.0}} ("Stimulators")) -> ()  [unwired: 2 in, 2 out]
        n114 = call <extravilib>:"Write.vi"("element"=w205) -> ("channel"=w202:T33)  [unwired: 8 in, 2 out]
      }
      event Value Change {
        w228 = T28."Enabled" ("Disabled")
        n115 = event-data() -> ()  [unwired: 1 in, 1 out]
        n116 = property on="Subject Parameters Folder" class="Path"() -> ("Value"=w242:path)  [unwired: 2 in, 2 out]
        n117 = Bundle By Name(cluster=w244, "Subject"="Subject") -> (w241:T39)
        n118 = call "Latest Parameters.vi"("Subject Number"="Subject", "Subject Parameters Folder"=w242) -> ("error in (no error)"=w239:errorcluster, "Subject Parameters"=w237:T22, "Source Parameter File"=w238:path)  [unwired: 2 in, 1 out]
        n119 = case shown="Error .." w239 {
          tunnel: w238 -> [w247 _]
          tunnel: w237 -> [w248 _]
          tunnel: [w248 w249] -> w235
          tunnel: [w247 w252] -> w226
          tunnel: [TRUE ("Value") TRUE ("Value")] -> w236
          frame No Error {
          }
          frame Error {
            n120 = call "Load Default Parameters.vi"("Default parameters file"="Local Default Parameters File") -> ("Subject Parameters"=w249:T22, "Subject Parameters File"=w252:path)  [unwired: 3 in]
            n121 = One Button Dialog(message="Parameters not found. Loading default parameters.") -> ()  [unwired: 1 in, 1 out]
          }
        }
        n122 = Bundle By Name(cluster=w241, "Subject Parameter File"=w226, "Subject Parameters"=w235) -> (w240:T39)
        n123 = Unbundle By Name(w235) -> ("Left GPD Params"=w234:T17, "Right GPD Params"=w233:T17, "Left Stim Params"=w231:T19, "Right Stim Params"=w230:T19)
        n124 = property on="Parameters Loaded?" class="Bool (strict)"("Value"=w236) -> ()  [unwired: 2 in, 2 out]
        n125 = Strip Path(path=w226) -> (name=→"Parameters File" →"Parameters File":string)  [unwired: 1 out]
        n126 = Bundle("Left GPD Params"=w234, "Right GPD Params"=w233) -> (→"GPD Params Display":T18)  [unwired: 1 in]
        n127 = Bundle("Left Stim Params"=w231, "Right Stim Params"=w230) -> (→"Stim Params Display":T21)  [unwired: 1 in]
        n128 = property on="View Edit Params" class="Bool"("DisabledEnum"=w228) -> ()  [unwired: 2 in, 2 out]
        n129 = property on="Start GPD" class="Bool"("DisabledEnum"=T28."Enabled" ("Disabled")) -> ()  [unwired: 2 in, 2 out]
        n130 = property on="Param Ctrls" class="Clust"("DisabledEnum"=w228) -> ()  [unwired: 2 in, 2 out]
        n131 = property on="Thresholding" class="Bool"("DisabledEnum"=w228) -> ()  [unwired: 2 in, 2 out]
      }
      event "Param Ctrls.Param Ctrls.Load Last Parameters", "Param Ctrls.Param Ctrls.Load Alternate Parameters", "Param Ctrls.Param Ctrls.Load Default Parameters": Value Change {
        n132 = event-data() -> ("CtlRef"=w264:refnum<vi>)  [unwired: 1 in]
        n133 = Unbundle By Name(w259) -> ("Subject"=w257:u16)
        n134 = property class="Bool"(reference=w264) -> ("Label.Text"=w263:string)  [unwired: 1 in, 2 out]
        n135 = property on="Local Default Parameters File" class="Path"() -> ("Value"=w256:path)  [unwired: 2 in, 2 out]
        n136 = call "Load Subject Parameters.vi"("Default Parameters File"=w256, "Subject"=w257, "Label.Text"=w263, "Subject Parameters Folder"="Subject Parameters Folder") -> ("Subject Parameters"=w258:T22, "Source Parameter File"=w255:path)  [unwired: 1 in, 1 out]
        "Source Parameter File" <- w255
        n137 = Strip Path(path=w255) -> (name=w254:string)  [unwired: 1 out]
        n138 = property on="Parameters File" class="Str"("Value"=w254) -> ()  [unwired: 2 in, 2 out]
        n139 = property on="Parameters File" class="Str"("Value"=w254) -> ()  [unwired: 2 in, 2 out]
        n140 = Bundle By Name(cluster=w259, "Subject Parameters"=w258) -> (w260:T39)
      }
      event "View Edit Params": Value Change {
        n141 = event-data() -> ()  [unwired: 1 in, 1 out]
        n142 = Unbundle By Name(w269) -> ("Subject Parameters"=w267:T22)
        n143 = call "View Edit Parameters.vi"("Subject Parameters In"=w267) -> ("Subject Parameters Out"=w266:T22)
        n144 = Bundle By Name(cluster=w269, "Subject Parameters"=w266) -> (w268:T39)
      }
      event "Thresholding": Value Change {
        n145 = event-data() -> ()  [unwired: 1 in, 1 out]
        n146 = call "CP FES Thresholding.vi"("CP FES Walking Data"=w271) -> ("CP FES Walking Data Out"=w270:T39)  [unwired: 2 in]
      }
      event Value Change {
        n147 = event-data() -> ()  [unwired: 1 in, 1 out]
        n148 = Bundle By Name(cluster=w275, "Stimulator Controls"="Stimulators") -> (w274:T39)
      }
      event Value Change {
        w281 = T31 {"Message"=enum."Initialize", "Data"=variant}  # Timer Messages
        n149 = event-data() -> ()  [unwired: 1 in, 1 out]
        n150 = property on="Protocol" class="Clust (strict)"() -> ("Value"=w278:T8)  [unwired: 2 in, 2 out]
        n151 = Bundle By Name(cluster=w284, "Protocol"=w278) -> (w283:T39)
        n152 = Unbundle By Name(w278) -> ("Protocol"=w279:T10)
        n153 = Bundle By Name(cluster=w281, "Data"=w279) -> (w280:T31)
        n154 = call <extravilib>:"Write.vi"("element"=w280) -> ("channel"=w277:T33)  [unwired: 8 in, 2 out]
      }
      event "Start GPD": Value Change {
        w301 = T26 {"State"=enum."Initialize", "Data"=variant}  # CP FES Message
        w303 = T28."Disabled and Grayed Out" ("Disabled")
        # "Call target VI asynchronously and forget"
        n155 = event-data() -> ()  [unwired: 1 in, 1 out]
        n156 = Unbundle By Name(w285) -> ("Subject Parameter File"=w290:path, "Stim Protocol Log File"=w289:path, "Protocol.Protocol"=w292:T10, "Current Interval Idx"=w291:i32, "Stimulator Controls"=w288, "Protocol.Protocol"=w286:T10, "Current Interval Idx"=w287:i32)
        n157 = property on="Start Timer" class="Bool"("DisabledEnum"=T28."Enabled" ("Disabled")) -> ()  [unwired: 2 in, 2 out]
        n158 = Index Array(array=w292, index=w291) -> (element=w293:T11)
        n159 = vi-ref "CP FES GPD and Stim.vi"() -> (w298:refnum<vi>)
        n160 = Bundle By Name(cluster=T38 {"Subject Parameter File"=path "", "Current Interval"={"Interval Type"=enum."Walk", "Duration"=20.0, " Mode"=enum."Stim", "Alt Period"=0.0}, "Stim Protocol Log File"=path ""} ("input cluster"), "Subject Parameter File"=w290, "Stim Protocol Log File"=w289, "Current Interval"=w293) -> (w300:T38)
        n161 = property class="VI"(reference=w298) -> ("Name"=w307:string)  [unwired: 1 in, 2 out]
        n162 = Open VI Reference(type specifier VI Refnum (for type only)=refnum<vi> refnum, vi path=w307, options=128) -> (vi reference=w296:refnum<vi>, error out=w294:errorcluster)  [unwired: 3 in]
        n163 = Bundle By Name(cluster=w301, "Data"=w300) -> (w305:T26)
        n164 = property on="Reset" class="Bool"("DisabledEnum"=w303) -> ()  [unwired: 2 in, 2 out]
        n165 = property on="Start GPD" class="Bool"("DisabledEnum"=w303) -> ()  [unwired: 2 in, 2 out]
        n166 = Enqueue Element(queue=w310, element=w305) -> (queue out=w295:refnum<queue>)  [unwired: 2 in, 2 out]
        n167 = property on="Manual Stim" class="Bool (strict)"("DisabledEnum"=w303) -> ()  [unwired: 2 in, 2 out]
        n168 = call-by-ref "Start Asynchronous Call"(reference=w296, error in=w294, "Stimulator Controls"=w288, "Message from Above"=w295) -> (reference out=w308:refnum<vi>, error out=w309:errorcluster)  [unwired: 8 in]
        n169 = case shown="0, Default" w287 {
          selector: w287 -> [_ w316]
          tunnel: w286 -> [w311 w315]
          frame 0, Default {
            # "First interval - initialize the timer"
            n170 = disable-structure shown="Disabled" {
              disable-tunnel: w311 -> [w312 _]
              frame Disabled {
                w314 = T31 {"Message"=enum."Initialize", "Data"=variant}  # Timer Messages
                n171 = Bundle By Name(cluster=w314, "Data"=w312) -> (w313:T31)
                n172 = call <extravilib>:"Write.vi"("element"=w313) -> ()  [unwired: 8 in, 3 out]
              }
              frame Enabled {
              }
            }
          }
          frame 1.. {
            # "Subsequent interval - resume on \"Start\""
            n173 = disable-structure shown="Disabled" {
              disable-tunnel: w316 -> [w319 _]
              disable-tunnel: w315 -> [w318 _]
              frame Disabled {
                w320 = T31 {"Message"=enum."Resume", "Data"=variant}  # Timer Messages
                n174 = Index Array(array=w318, index=w319) -> (element=w321:T11)
                n175 = Bundle By Name(cluster=w320, "Data"=w321) -> (w317:T31)
                n176 = call <extravilib>:"Write.vi"("element"=w317) -> ()  [unwired: 8 in, 3 out]
              }
              frame Enabled {
              }
            }
          }
        }
        n177 = property on="Pause" class="Bool (strict)"("DisabledEnum"=w303) -> ()  [unwired: 2 in, 2 out]
        n178 = Close Reference(reference=w308, error in (no error)=w309) -> ()  [unwired: 1 out]
      }
      event "Start Timer": Value Change {
        w325 = T26 {"State"=enum."Start Timer", "Data"=variant}  # CP FES Message
        w327 = T28."Enabled" ("Disabled")
        w328 = T28."Disabled and Grayed Out" ("Disabled")
        n179 = event-data() -> ()  [unwired: 1 in, 1 out]
        n180 = Unbundle By Name(w322) -> ("Current Interval Idx"=w323:i32)
        n181 = Enqueue Element(queue=w324, element=w325) -> ()  [unwired: 2 in, 3 out]
        n182 = property on="Stop" class="Bool"("DisabledEnum"=w327) -> ()  [unwired: 2 in, 2 out]
        n183 = property on="Pause" class="Bool (strict)"("DisabledEnum"=w327) -> ()  [unwired: 2 in, 2 out]
        n184 = case shown="0, Default" w323 {
          tunnel: [w331 w332] -> w329
          frame 0, Default {
            w331 = T31 {"Message"=enum."Start", "Data"=variant}  # Timer Messages
          }
          frame 1.. {
            w332 = T31 {"Message"=enum."Resume", "Data"=variant}  # Timer Messages
          }
        }
        n185 = property on="Start Timer" class="Bool"("DisabledEnum"=w328) -> ()  [unwired: 2 in, 2 out]
        n186 = property on="Manual Stim" class="Bool (strict)"("DisabledEnum"=w328) -> ()  [unwired: 2 in, 2 out]
        n187 = call <extravilib>:"Write.vi"("element"=w329) -> ("channel"=w330:T33)  [unwired: 8 in, 2 out]
      }
      event "Pause": Value Change {
        w338 = T28."Enabled" ("Disabled")
        w337 = T28."Disabled and Grayed Out" ("Disabled")
        n188 = event-data() -> ()  [unwired: 1 in, 1 out]
        n189 = case shown="True" "Pause" {
          tunnel: [w344 w348] -> w339
          tunnel: [w342 w345] -> w336
          frame False {
            w342 = T31 {"Message"=enum."Resume", "Data"=variant}  # Timer Message
            w344 = T26 {"State"=enum."Resume", "Data"=variant}  # GPD Messages
            # "Pause to Resume"
            n190 = property on="Reset" class="Bool"("DisabledEnum"=T28."Disabled and Grayed Out" ("Disabled")) -> ()  [unwired: 2 in, 2 out]
          }
          frame True {
            w345 = T31 {"Message"=enum."Pause", "Data"=variant}  # Timer Message
            w348 = T26 {"State"=enum."Pause", "Data"=variant}  # GPD Messages
            # "On to Pause"
            n191 = property on="Start Timer" class="Bool"("DisabledEnum"=T28."Disabled and Grayed Out" ("Disabled")) -> ()  [unwired: 2 in, 2 out]
            n192 = property on="Reset" class="Bool"("DisabledEnum"=T28."Enabled" ("Disabled")) -> ()  [unwired: 2 in, 2 out]
          }
        }
        n193 = Enqueue Element(queue=w341, element=w339) -> ()  [unwired: 2 in, 3 out]
        n194 = call <extravilib>:"Write.vi"("element"=w336) -> ("channel"=w335:T33)  [unwired: 8 in, 2 out]
        n195 = property on="Start GPD" class="Bool"("DisabledEnum"=w337) -> ()  [unwired: 2 in, 2 out]
        n196 = property on="Manual Stim" class="Bool (strict)"("DisabledEnum"=w337) -> ()  [unwired: 2 in, 2 out]
        n197 = property on="Stop" class="Bool"("DisabledEnum"=w338) -> ()  [unwired: 2 in, 2 out]
        n198 = property on="Pause" class="Bool (strict)"("DisabledEnum"=w338) -> ()  [unwired: 2 in, 2 out]
      }
      event "Reset": Value Change {
        w350 = T26 {"State"=enum."Reset", "Data"=variant}  # GPD Messages
        w356 = T31 {"Message"=enum."Reset", "Data"=variant}  # Timer Messages
        n199 = event-data() -> ()  [unwired: 1 in, 1 out]
        n200 = Enqueue Element(queue=w351, element=w350) -> ()  [unwired: 2 in, 3 out]
        n201 = property on="Reset" class="Bool"("Value"=FALSE ("Reset"), "DisabledEnum"=T28."Disabled and Grayed Out" ("Disabled")) -> ()  [unwired: 2 in, 2 out]
        n202 = call <extravilib>:"Write.vi"("element"=w356) -> ("channel"=w355:T33)  [unwired: 8 in, 2 out]
      }
      event "Stop": Value Change {
        w359 = T31 {"Message"=enum."Stop", "Data"=variant}  # Timer Messages
        w362 = T26 {"State"=enum."Stop", "Data"=variant}  # GPD Messages
        n203 = event-data() -> ()  [unwired: 1 in, 1 out]
        n204 = Enqueue Element(queue=w361, element=w362) -> ()  [unwired: 2 in, 3 out]
        n205 = call <extravilib>:"Write.vi"("element"=w359) -> ("channel"=w358:T33)  [unwired: 8 in, 2 out]
      }
      event "Manual Stim": Value Change {
        # "Run target VI and wait for user to close it"
        n206 = event-data() -> ()  [unwired: 1 in, 1 out]
        n207 = flat-sequence {
          tunnel: [w371] -> w367
          tunnel: w366 -> [w371]
          tunnel: w363 -> [w370]
          tunnel: [w370] -> w365
          tunnel: [w369] -> w364
          tunnel: w367 -> [w379]
          tunnel: w365 -> [w375]
          tunnel: w364 -> [w373]
          frame #0 {
            w372 = T28."Disabled and Grayed Out" ("Disabled")
            n208 = property on="Manual Stim" class="Bool (strict)"("DisabledEnum"=w372) -> ()  [unwired: 2 in, 2 out]
            n209 = property on="Start Timer" class="Bool"("DisabledEnum"=w372) -> ()  [unwired: 2 in, 2 out]
            n210 = property on="Pause" class="Bool (strict)"("DisabledEnum"=w372) -> ()  [unwired: 2 in, 2 out]
            n211 = Unbundle By Name(w370) -> ("Subject"=w369:u16)
            n212 = property on="Start GPD" class="Bool"("DisabledEnum"=w372) -> ()  [unwired: 2 in, 2 out]
            n213 = property on="Stop" class="Bool"("DisabledEnum"=w372) -> ()  [unwired: 2 in, 2 out]
            n214 = property on="Reset" class="Bool"("DisabledEnum"=w372) -> ()  [unwired: 2 in, 2 out]
          }
          frame #1 {
            n215 = Unbundle By Name(w375) -> ("Stimulator Controls"=w374)
            n216 = Bundle By Name(cluster=T26 {"State"=enum."Manual", "Data"=variant} ("element"), "Data"=w373) -> (w376:T26)
            n217 = Enqueue Element(queue=w379, element=w376) -> (queue out=w378:refnum<queue>)  [unwired: 2 in, 2 out]
            n218 = call "CP FES GPD and Stim.vi"("Stimulator Controls"=w374, "Message from Above"=w378) -> ()  [unwired: 8 in]
          }
          frame #2 {
            w380 = T28."Enabled" ("Disabled")
            n219 = property on="Stop" class="Bool"("DisabledEnum"=w380) -> ()  [unwired: 2 in, 2 out]
            n220 = property on="Start GPD" class="Bool"("DisabledEnum"=w380) -> ()  [unwired: 2 in, 2 out]
            n221 = property on="Manual Stim" class="Bool (strict)"("DisabledEnum"=w380, "Value"=FALSE ("Manual Stim")) -> ()  [unwired: 2 in, 2 out]
          }
        }
      }
      event "Stop GPD": Value Change {
        w385 = T26 {"State"=enum."Stop", "Data"=variant}  # GPD Messages
        n222 = event-data() -> ()  [unwired: 1 in, 1 out]
        n223 = Enqueue Element(queue=w384, element=w385) -> ()  [unwired: 2 in, 3 out]
      }
      event User Event {
        w388 = T26 {"State"=enum."Stop", "Data"=variant}  # GPD Messages
        # "Timer has reached the end of the session. Stop the event loop (state machine loop is already stopped) and send \"Stop\" message to the target VI."
        n224 = event-data() -> ()  [unwired: 1 in, 1 out]
        n225 = Enqueue Element(queue=w387, element=w388) -> ()  [unwired: 2 in, 3 out]
      }
      event User Event {
        w395 = T28."Enabled" ("Disabled")
        w396 = T31 {"Message"=enum."Pause", "Data"=variant}  # Timer Message
        w394 = T28."Disabled and Grayed Out" ("Disabled")
        n226 = event-data() -> ()  [unwired: 1 in, 1 out]
        n227 = Unbundle By Name(w391) -> ("Current Interval Idx"=w393:i32)
        n228 = property on="Start Timer" class="Bool"("DisabledEnum"=w394) -> ()  [unwired: 2 in, 2 out]
        n229 = property on="Pause" class="Bool (strict)"("DisabledEnum"=w394) -> ()  [unwired: 2 in, 2 out]
        n230 = property on="Start GPD" class="Bool"("DisabledEnum"=w395) -> ()  [unwired: 2 in, 2 out]
        n231 = property on="Manual Stim" class="Bool (strict)"("DisabledEnum"=w395) -> ()  [unwired: 2 in, 2 out]
        n232 = Increment(x=w393) -> (x+1=w392:i32)
        n233 = Bundle By Name(cluster=w391, "Current Interval Idx"=w392) -> (w390:T39)
        n234 = call <extravilib>:"Write.vi"("element"=w396) -> ("channel"=w397:T33)  [unwired: 8 in, 2 out]
      }
    }
  }
  n235 = while "Timer State Machine" {
    tunnel: w2 -> [w415]
    tunnel: w2 -> [w413]
    shift-right: [w403] -> _
    shift-left: _ -> [w405]
    tunnel: [w412] -> w4
    tunnel: w1 -> [w411]
    tunnel: [w410] -> _
    tunnel: [w409] -> w3
    shift-right: [w404] -> _
    shift-left: 0 ("timeout in ms (-1)") -> [w406]
    stop <- w414 stop-if-true
    # "Add message to update display"
    n236 = call <extravilib>:"Read.vi"("timeout in ms (-1)"=w406, "channel"=w415) -> ("element"=w408:T31, "timedout?"=w407:bool)  [unwired: 6 in, 2 out]
    n237 = case shown="True" w407 {
      tunnel: [w428 FALSE] -> w414
      tunnel: [w427 w506] -> w413
      tunnel: [w426 _] -> w412
      tunnel: w411 -> [w425 w513]
      tunnel: [w424 w507] -> w410
      tunnel: [w423 _] -> w409
      tunnel: [w422 w515] -> w403
      tunnel: w408 -> [w419 _]
      tunnel: w405 -> [w418 w510]
      tunnel: [w420 w509] -> w404
      frame False {
        # "Message received - process message"
        n238 = Unbundle By Name(w419) -> ("Data"=w421:variant, "Message"=w417:T32)
        n239 = Bundle By Name(cluster=w418, "Protocol Timer State"=w417) -> (w416:T29)
        n240 = case shown="\"Reset\"" w417 {
          tunnel: [FALSE FALSE FALSE FALSE FALSE FALSE FALSE w494 FALSE] -> w428
          tunnel: w421 -> [w443 _ _ _ _ _ w489 _ _]
          tunnel: [_ _ _ _ w464 w476 _ _ w503] -> w427
          tunnel: w416 -> [w441 w446 w449 w454 w463 w473 w486 w495 w505]
          tunnel: [w440 w446 w449 w454 w462 w471 w485 w495 w504] -> w422
          tunnel: [_ _ _ _ _ _ _ w493 _] -> w426
          tunnel: w425 -> [w438 w445 w448 w453 w461 w470 w480 w492 w501]
          tunnel: [w438 w445 w448 w453 w461 w470 w480 w492 w501] -> w424
          tunnel: [_ _ _ _ _ _ w481 _ _] -> w423
          tunnel: [-1 ("timeout in ms (-1)") -1 ("timeout in ms (-1)") 0 ("timeout in ms (-1)") -1 ("timeout in ms (-1)") -1 ("timeout in ms (-1)") -1 ("timeout in ms (-1)") -1 ("timeout in ms (-1)") -1 ("timeout in ms (-1)") -1 ("timeout in ms (-1)")] -> w420
          frame "Initialize" {
            w437 = T11[] []  # Protocol type
            # "Wait for message"
            n241 = Variant To Data(type=w437, Variant=w443) -> (data=w435:T11[])  [unwired: 1 in, 1 out]
            n242 = call "Compute Protocol Duration.vi"("Protocol"=w435) -> ("Protocol Duration (s)"=w430:dbl[unit])  [unwired: 3 in, 1 out]
            n243 = Index Array(array=w435, index=0) -> (element=w436:T11)
            n244 = call "Initialize Current Interval Indicator.vi"("Protocol"=w435) -> ("Current Interval Indicator"=w439:bool[])  [unwired: 2 in]
            n245 = call "Get Interval Duration.vi"("Interval"=w436) -> ("Interval Duration (s)"=w429:dbl[unit])  [unwired: 3 in, 1 out]
            n246 = Bundle By Name(cluster=w441, "Curent interval duration"=w429, "Time to next interval"=w429, "Remaining session time"=w430, "Current interval indicator"=w439, "Current interval index"=u32 0, "Time elapsed in current iteration"=dbl[unit] 0.0, "Protocol"=w435) -> (w440:T29)
          }
          frame "Idle", Default {
          }
          frame "On" {
            # "Timeout to default (see \"True\" case)"
          }
          frame "Pause" {
          }
          frame "Resume" {
            w465 = T31 {"Message"=enum."On", "Data"=variant}  # Timer Message
            # "Could just update \"Timer State\" to \"On\" but this is more\nconsistent with state machine paradigm"
            n247 = Tick Count (ms) "Current time"() -> (millisecond timer value=w458:u32)
            n248 = To Double Precision Float(number=w458) -> (double precision float=w457:dbl)
            n249 = Divide(x=w457, y=dbl[unit] 1000.0) -> (x/y=w456:dbl[unit])
            n250 = Bundle By Name(cluster=w463, "Time of last iteration"=w456) -> (w462:T29)
            n251 = call <extravilib>:"Write.vi"("element"=w465) -> ("channel"=w464:T33)  [unwired: 8 in, 2 out]
          }
          frame "Reset" {
            w477 = T31 {"Message"=enum."Pause", "Data"=variant}  # Timer Messages
            n252 = Unbundle By Name(w473) -> ("Curent interval duration"=w469:dbl[unit], "Remaining session time"=w475:dbl[unit], "Time elapsed in current iteration"=w474:dbl[unit])
            n253 = Add(x=w475, y=w474) -> (x+y=w472:dbl[unit])
            n254 = Bundle By Name(cluster=w473, "Time to next interval"=w469, "Remaining session time"=w472, "Time elapsed in current iteration"=dbl[unit] 0.0) -> (w471:T29)
            n255 = call <extravilib>:"Write.vi"("element"=w477) -> ("channel"=w476:T33)  [unwired: 8 in, 2 out]
          }
          frame "Transition" {
            w490 = T11 {"Interval Type"=enum."Walk", "Duration"=20.0, " Mode"=enum."Stim", "Alt Period"=0.0}  # Interval data type
            # "To go into pause state? Why not\njust transition into pause?"
            # "Interval Over dynamic event"
            n256 = Variant To Data(type=w490, Variant=w489) -> (data=w483:T11)  [unwired: 1 in, 1 out]
            n257 = Unbundle By Name(w483) -> ("Duration"=w488:dbl[unit])
            n258 = Bundle By Name(cluster=w486, "Time elapsed in current iteration"=dbl[unit] 0.0, "Time to next interval"=w488, "Curent interval duration"=w488) -> (w485:T29)
            n259 = call <extravilib>:"Write.vi"("element"=TRUE) -> ("channel"=w481:T34)  [unwired: 9 in, 1 out]
          }
          frame "Stop" {
            w494 = TRUE
            n260 = call <extravilib>:"Write.vi"("element"=w494) -> ("channel"=w493:T34)  [unwired: 9 in, 1 out]
          }
          frame "Start" {
            w502 = T31 {"Message"=enum."On", "Data"=variant}  # Timer Messages
            n261 = Tick Count (ms)() -> (millisecond timer value=w498:u32)
            n262 = Divide(x=w498, y=dbl[unit] 1000.0) -> (x/y=w496:dbl[unit])
            n263 = Bundle By Name(cluster=w505, "Time of last iteration"=w496) -> (w504:T29)
            n264 = call <extravilib>:"Write.vi"("element"=w502) -> ("channel"=w503:T33)  [unwired: 8 in, 2 out]
          }
        }
      }
      frame True {
        # "Timed out - default behavior"
        n265 = Unbundle By Name(w510) -> ("Current interval index"=w511:u32, "Protocol"=w512:T11[], "Protocol Timer State"=w514:T30)
        n266 = case "What state?" shown="\"Initialize\", Default" w514 {
          tunnel: [w518 w552] -> w515
          tunnel: w513 -> [w523 w553]
          tunnel: w512 -> [w522 _]
          tunnel: w511 -> [w521 _]
          tunnel: w510 -> [w520 _]
          tunnel: [5 ("timeout in ms (-1)") -1 ("timeout in ms (-1)")] -> w509
          tunnel: [w517 w553] -> w507
          tunnel: [w516 _] -> w506
          frame "Start" {
            # "5 ms increments"
            n267 = call "Update Timer Data.vi"("Timer Data for timer in"=w520) -> ("Interval up?"=w525:bool, "Timer Data for timer out"=w524:T29)  [unwired: 3 in]
            n268 = case "Interval over?" shown="True" w525 {
              tunnel: w521 -> [_ w536]
              tunnel: [_ w538] -> w516
              tunnel: w522 -> [_ w534]
              tunnel: w524 -> [w527 w533]
              tunnel: [w527 w532] -> w518
              tunnel: w523 -> [w526 w530]
              tunnel: [w526 w529] -> w517
              frame False {
                # "Keep goin'!"
              }
              frame True {
                w531 = T26 {"State"=enum."Stim Off", "Data"=variant}  # CP FES Message
                n269 = Increment(x=w536) -> (x+1=w528:u32)
                n270 = Array Size(array=w534) -> (size(s)=w537:i32)
                n271 = Equal?(x=w528, y=w537) -> (x = y?=w535:bool)
                n272 = case "Session Over?" shown="False" w535 {
                  tunnel: w536 -> [w540 _]
                  tunnel: [w548 w551] -> w538
                  tunnel: w534 -> [w544 _]
                  tunnel: w533 -> [w543 w549]
                  tunnel: [w542 w549] -> w532
                  frame False {
                    w547 = T31 {"Message"=enum."Transition", "Data"=variant}  # Timer Messages
                    # "Get next interval"
                    # "Advance to next interval"
                    n273 = Increment(x=w540) -> (x+1=w539:u32)
                    n274 = call "Update Current Interval Indicator.vi"("Interval idx"=w544, "Protocol.Active Interval"=w539) -> ("Protocol.Active Interval"=w541:bool[])  [unwired: 3 in]
                    n275 = Bundle By Name(cluster=w543, "Current interval index"=w539, "Current interval indicator"=w541) -> (w542:T29)
                    n276 = Index Array(array=w544, index=w539) -> (element=w545:T11)
                    n277 = Bundle By Name(cluster=w547, "Data"=w545) -> (w546:T31)
                    n278 = call <extravilib>:"Write.vi"("element"=w546) -> ("channel"=w548:T33)  [unwired: 8 in, 2 out]
                  }
                  frame True {
                    w550 = T31 {"Message"=enum."Stop", "Data"=variant}  # Timer Messages
                    # "We're done!"
                    n279 = call <extravilib>:"Write.vi"("element"=w550) -> ("channel"=w551:T33)  [unwired: 8 in, 2 out]
                  }
                }
                n280 = Enqueue Element(queue=w530, element=w531) -> (queue out=w529:refnum<queue>)  [unwired: 2 in, 2 out]
              }
            }
          }
          frame "Initialize", Default {
            w552 = T29 {"Protocol Timer State"=enum."Initialize", "Remaining session time"=0.0, "Curent interval duration"=0.0, "Time of last iteration"=0.0, "Time elapsed in current iteration"=0.0, "Current interval indicator"=[], "Current interval index"=0, "Time to next interval"=0.0, "Protocol"=[]}  # Timer Data for timer
            # "This is the \"Startup\" behavior"
            # "Wait for message"
          }
        }
      }
    }
    n281 = Unbundle By Name(w403) -> ("Protocol Timer State"=→"Timer State":T30, "Current interval indicator"=w399:bool[], "Remaining session time"=→"Session Time":dbl[unit], "Time to next interval"=→"Time to Next Interval":dbl[unit])
    n282 = property on="Active Interval" class="Arr (strict)"("Value"=w399) -> ()  [unwired: 2 in, 2 out]
  }
